vi "Main.vi"(11 "Module Admin":refnum<class "Delacor_lib_QMH_Cloneable Module Admin.lvclass">) -> ()   [LabVIEW 2020, in "NI DAQ.lvlib"]
doc: "This template is based off of the Queued Message Handler design pattern and the Queued Message Handler project template that ships with LabVIEW.\n\nThe main difference is that the queue is private to this module and communication between modules is performed via Broadcast and Request events.\n\nRequest events are wrapped in public API methods and are handled in the Event Handling Loop (EHL) of this VI. Any module can register for Broadcast events sent by this module. The EHL generates messages based on user interface actions.\n\nThe Message Handling Loop (MHL) processes messages generated by the EHL, or by other messages. The messages are string values, so new messages can be added easily to the Message Cases case structure in the MHL. Each message cluster can also provide an optional value for Message Data, which is a variant that can be converted to whatever message-specific data is required.\n_____\nBased on DQMH Project Template 6.1.0.94."
uses:
  NI DAQ.lvlib
  <vilib>/Delacor/Delacor QMH/Libraries/Cloneable Module Admin_class/Delacor_lib_QMH_Cloneable Module Admin.lvclass
  <vilib>/ErrorRing/Error Ring.xnode
  <vilib>/Delacor/Delacor QMH/Libraries/Message Queue_class/Delacor_lib_QMH_Message Queue.lvclass
  Module Data--cluster.ctl
  <vilib>/Utility/miscctls.llb/LVPointTypeDef.ctl
  <vilib>/Utility/error.llb/Error Cluster From Error Code.vi
  <vilib>/Delacor/Delacor QMH/Libraries/Message Queue_class/Delacor_lib_QMH_Enqueue Message (Single).vi
  Stop Argument--cluster.ctl
  Set device ID Argument--cluster.ctl
  Get channel list (Reply Payload)--cluster.ctl
  Get channel list Argument--cluster.ctl
  Start task Argument--cluster.ctl
  Stop task Argument--cluster.ctl
  Write DO Argument--cluster.ctl
  Create DI channel Argument--cluster.ctl
  Read DI (Reply Payload)--cluster.ctl
  Read DI Argument--cluster.ctl
  Support/Task list.ctl
  Get task ref (Reply Payload)--cluster.ctl
  Get task ref Argument--cluster.ctl
  <vilib>/DAQmx/write.llb/DAQmx Write (Digital 1D Bool 1Chan 1Samp).vi
  Create AI channel Argument--cluster.ctl
  Read AI (Reply Payload)--cluster.ctl
  Read AI Argument--cluster.ctl
  Create AO channel Argument--cluster.ctl
  AI config parameters--cluster.ctl
  Write AO Argument--cluster.ctl
  Validate connection Argument--cluster.ctl
  <resource>/objmgr/daqmx.rc
  Validate connection (Reply Payload)--cluster.ctl
  <vilib>/DAQmx/write.llb/DAQmx Write (Digital Bool 1Line 1Point).vi
  <vilib>/DAQmx/write.llb/DAQmx Write (Analog DBL 1Chan 1Samp).vi
  <vilib>/DAQmx/read.llb/DAQmx Read (Analog 1D DBL NChan 1Samp).vi
  <vilib>/DAQmx/read.llb/DAQmx Read (Analog DBL 1Chan 1Samp).vi
  <vilib>/DAQmx/create/channels.llb/DAQmx Create Channel (DO-Digital Output).vi
  <vilib>/DAQmx/create/channels.llb/DAQmx Create Channel (AI-Voltage-Basic).vi
  <vilib>/DAQmx/create/channels.llb/DAQmx Create Channel (DI-Digital Input).vi
  <vilib>/DAQmx/write.llb/DAQmx Write (Analog 1D DBL NChan 1Samp).vi
  Support/Continuous aquisition params.ctl
  Start continous acquisition Argument--cluster.ctl
  Stop continuous acquisition Argument--cluster.ctl
  <vilib>/DAQmx/write.llb/DAQmx Write (Digital 1D Bool NChan 1Samp 1Line).vi
  <vilib>/DAQmx/read.llb/DAQmx Read (Digital 1D Bool 1Chan 1Samp).vi
  <vilib>/DAQmx/read.llb/DAQmx Read (Digital 1D Bool NChan 1Samp 1Line).vi
  Create DO channel Argument--cluster.ctl
  Create CI channel Argument--cluster.ctl
  <vilib>/DAQmx/create/channels.llb/DAQmx Create Channel (CI-Count Edges).vi
  <vilib>/DAQmx/create/channels.llb/DAQmx Create Channel (AO-Voltage-Basic).vi
  Read CI (Reply Payload)--cluster.ctl
  Read CI Argument--cluster.ctl
  <vilib>/DAQmx/read.llb/DAQmx Read (Counter DBL 1Chan 1Samp).vi
  <vilib>/DAQmx/read.llb/DAQmx Read (Counter 1D DBL NChan 1Samp).vi
  <vilib>/DAQmx/read.llb/DAQmx Read (Digital Bool 1Line 1Point).vi
  <vilib>/DAQmx/read.llb/DAQmx Read (Digital 1D U8 1Chan NSamp).vi
panel:
  out "error out":errorcluster
  out "Status":string
  in  "Simulate EHL Error":bool
  in  "Simulate MHL Error":bool
  # "Other QMH Modules communicate with this Module via its Public API (wrappers for its Request Events).\n\nThis Module communicates with other Modules via its Broadcast Events.\nAny module that wants to get these messages, just registers for this module's Broadcast events."
  # "This template is for the Delacor Modified Queued Message Handler design pattern.\n\nSee the block diagram for more information on how to use this template."
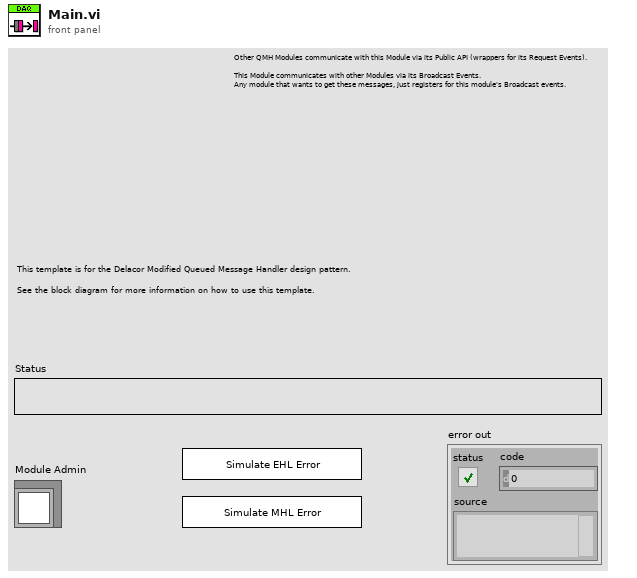
[diagram p1: front panel]
types:
  T1 = typedef "NI DAQ.lvlib/Request Events--cluster.ctl" = cluster{"Stop Module":refnum<user-event>, "Show Panel":refnum<user-event>, "Hide Panel":refnum<user-event>, "Show Diagram":refnum<user-event>, "Get Module Execution Status":refnum<user-event>, "Set device ID":refnum<user-event>, "Get channel list":refnum<user-event>, "Start task":refnum<user-event>, "Stop task":refnum<user-event>, "Write DO":refnum<user-event>, "Create DI channel":refnum<user-event>, "Read DI":refnum<user-event>, "Get task ref":refnum<user-event>, "Wake up HL":refnum<user-event>, "Sleep HL":refnum<user-event>, "Create AI channel":refnum<user-event>, "Read AI":refnum<user-event>, "Create AO channel":refnum<user-event>, "Write AO":refnum<user-event>, "Validate connection":refnum<user-event>, "Start continous acquisition":refnum<user-event>, "Stop continuous acquisition":refnum<user-event>, "Create DO channel":refnum<user-event>, "Create CI channel":refnum<user-event>, "Read CI":refnum<user-event>}
  T2 = cluster{"Wake HL":refnum<user-event>, "Sleep HL":refnum<user-event>}
  T3 = typedef "NI DAQ.lvlib/Continuous aquisition params.ctl" = cluster{"Module ID":i32, "Task list":T4, "Timeout":i32, "Acq type":enum16{"Single", "Multiple"}, "Data in":variant, "DAQmx Task":refnum<k21>, "N samples":i32}
  T4 = typedef "NI DAQ.lvlib/Task list.ctl" = enum16{"All", "DO task", "DI task", "AO task", "AI task", "CI task", "CO task"}
  T5 = typedef "NI DAQ.lvlib/Module Data--cluster.ctl" = cluster{"Status":string, "DO task":refnum<k21>, "DI task":refnum<k21>, "AO task":refnum<k21>, "AI task":refnum<k21>, "Device name":tag, "CI task":refnum<k21>, "CO task":refnum<k21>}
  T6 = enum32{"invalid lock state", "Not Locked", "Locked (No Password)", "Password-protected"}
  T7 = typedef "NI DAQ.lvlib/Stop Argument--cluster.ctl" = cluster{"Module ID":i32, "Origin":string, "Exit via Stop Module Req?":bool, "Wait for Module to stop?":bool}
  T8 = typedef "NI DAQ.lvlib/Set device ID Argument--cluster.ctl" = cluster{"Module ID":i32, "Device ID":tag}
  T9 = typedef "NI DAQ.lvlib/Get channel list Argument--cluster.ctl" = cluster{"Module ID":i32, "Wait Notifier":refnum<notifier>, "wait for reply":bool}
  T10 = typedef "NI DAQ.lvlib/Start task Argument--cluster.ctl" = cluster{"Module ID":i32, "Task list":T4}
  T11 = typedef "NI DAQ.lvlib/Stop task Argument--cluster.ctl" = cluster{"Module ID":i32, "Task list":T4}
  T12 = typedef "NI DAQ.lvlib/Write DO Argument--cluster.ctl" = cluster{"Module ID":i32, "Samples":enum16{"Single", "Multiple"}, "Data":bool[]}
  T13 = typedef "NI DAQ.lvlib/Create DI channel Argument--cluster.ctl" = cluster{"Module ID":i32, "Physical channel":string, "Channel name":string}
  T14 = typedef "NI DAQ.lvlib/Read DI Argument--cluster.ctl" = cluster{"Module ID":i32, "Samples":enum16{"Single", "Multiple"}, "Wait Notifier":refnum<notifier>, "wait for reply":bool}
  T15 = typedef "NI DAQ.lvlib/Get task ref Argument--cluster.ctl" = cluster{"Module ID":i32, "Task list":T4, "Wait Notifier":refnum<notifier>, "wait for reply":bool}
  T16 = typedef "NI DAQ.lvlib/Create AI channel Argument--cluster.ctl" = cluster{"Module ID":i32, "Physical channel":string, "Channel name":string, "Config params":cluster{"input terminal configuration":i32, "minimum value":dbl, "maximum value":dbl}}
  T17 = typedef "NI DAQ.lvlib/Read AI Argument--cluster.ctl" = cluster{"Module ID":i32, "Samples":enum16{"Single", "Multiple"}, "Wait Notifier":refnum<notifier>, "wait for reply":bool}
  T18 = typedef "NI DAQ.lvlib/Create AO channel Argument--cluster.ctl" = cluster{"Module ID":i32, "Physical channel":string, "Channel name":string, "Config params":T19}
  T19 = typedef "NI DAQ.lvlib/AI config parameters--cluster.ctl" = cluster{"Terminal configuration":i32, "min value":dbl, "max value":dbl}
  T20 = typedef "NI DAQ.lvlib/Write AO Argument--cluster.ctl" = cluster{"Module ID":i32, "Value(s)":dbl[], "Samples":enum16{"Single", "Multiple"}}
  T21 = typedef "NI DAQ.lvlib/Validate connection Argument--cluster.ctl" = cluster{"Module ID":i32, "Wait Notifier":refnum<notifier>, "wait for reply":bool}
  T22 = typedef "NI DAQ.lvlib/Start continous acquisition Argument--cluster.ctl" = cluster{"Module ID":i32, "Task list":T4, "Timeout":i32, "Acq type":enum16{"Single", "Multiple"}, "N samples":i32, "Data in":variant}
  T23 = typedef "NI DAQ.lvlib/Stop continuous acquisition Argument--cluster.ctl" = cluster{"Module ID":i32, "Boolean":bool}
  T24 = typedef "NI DAQ.lvlib/Create DO channel Argument--cluster.ctl" = cluster{"Module ID":i32, "lines":tag, "Channel name":string}
  T25 = typedef "NI DAQ.lvlib/Create CI channel Argument--cluster.ctl" = cluster{"Module ID":i32, "Physical channel":string, "Channel name":string, "Channel config":cluster{"Initial count":u32, "Count direction":i32, "Edge":i32}}
  T26 = typedef "NI DAQ.lvlib/Read CI Argument--cluster.ctl" = cluster{"Module ID":i32, "Samples":enum16{"Single", "Multiple"}, "Wait Notifier":refnum<notifier>, "wait for reply":bool}
  T27 = typedef "LVPointTypeDef.ctl" = cluster{"Horizontal":i16, "Vertical":i16}
  T28 = enum32{"Invalid", "Standard", "Closed", "Hidden", "Minimized", "Maximized"}
  T29 = typedef "NI DAQ.lvlib/Get channel list (Reply Payload)--cluster.ctl" = cluster{"Available channels":i32, "error":errorcluster, "Available channels 2":string[][]}
  T30 = typedef "NI DAQ.lvlib/Read DI (Reply Payload)--cluster.ctl" = cluster{"Data":bool[], "error":errorcluster}
  T31 = typedef "NI DAQ.lvlib/Read AI (Reply Payload)--cluster.ctl" = cluster{"Data":dbl[], "error":errorcluster}
  T32 = typedef "NI DAQ.lvlib/Get task ref (Reply Payload)--cluster.ctl" = cluster{"DAQmx Task":refnum<k21>, "error":errorcluster}
  T33 = typedef "NI DAQ.lvlib/Validate connection (Reply Payload)--cluster.ctl" = cluster{"DevSerialNum":u32, "error":errorcluster}
  T34 = typedef "NI DAQ.lvlib/Read CI (Reply Payload)--cluster.ctl" = cluster{"Module ID":i32, "data":dbl[], "error":errorcluster}
  T35 = cluster{"input terminal configuration":i32, "minimum value":dbl, "maximum value":dbl}
  T36 = cluster{"Initial count":u32, "Count direction":i32, "Edge":i32}
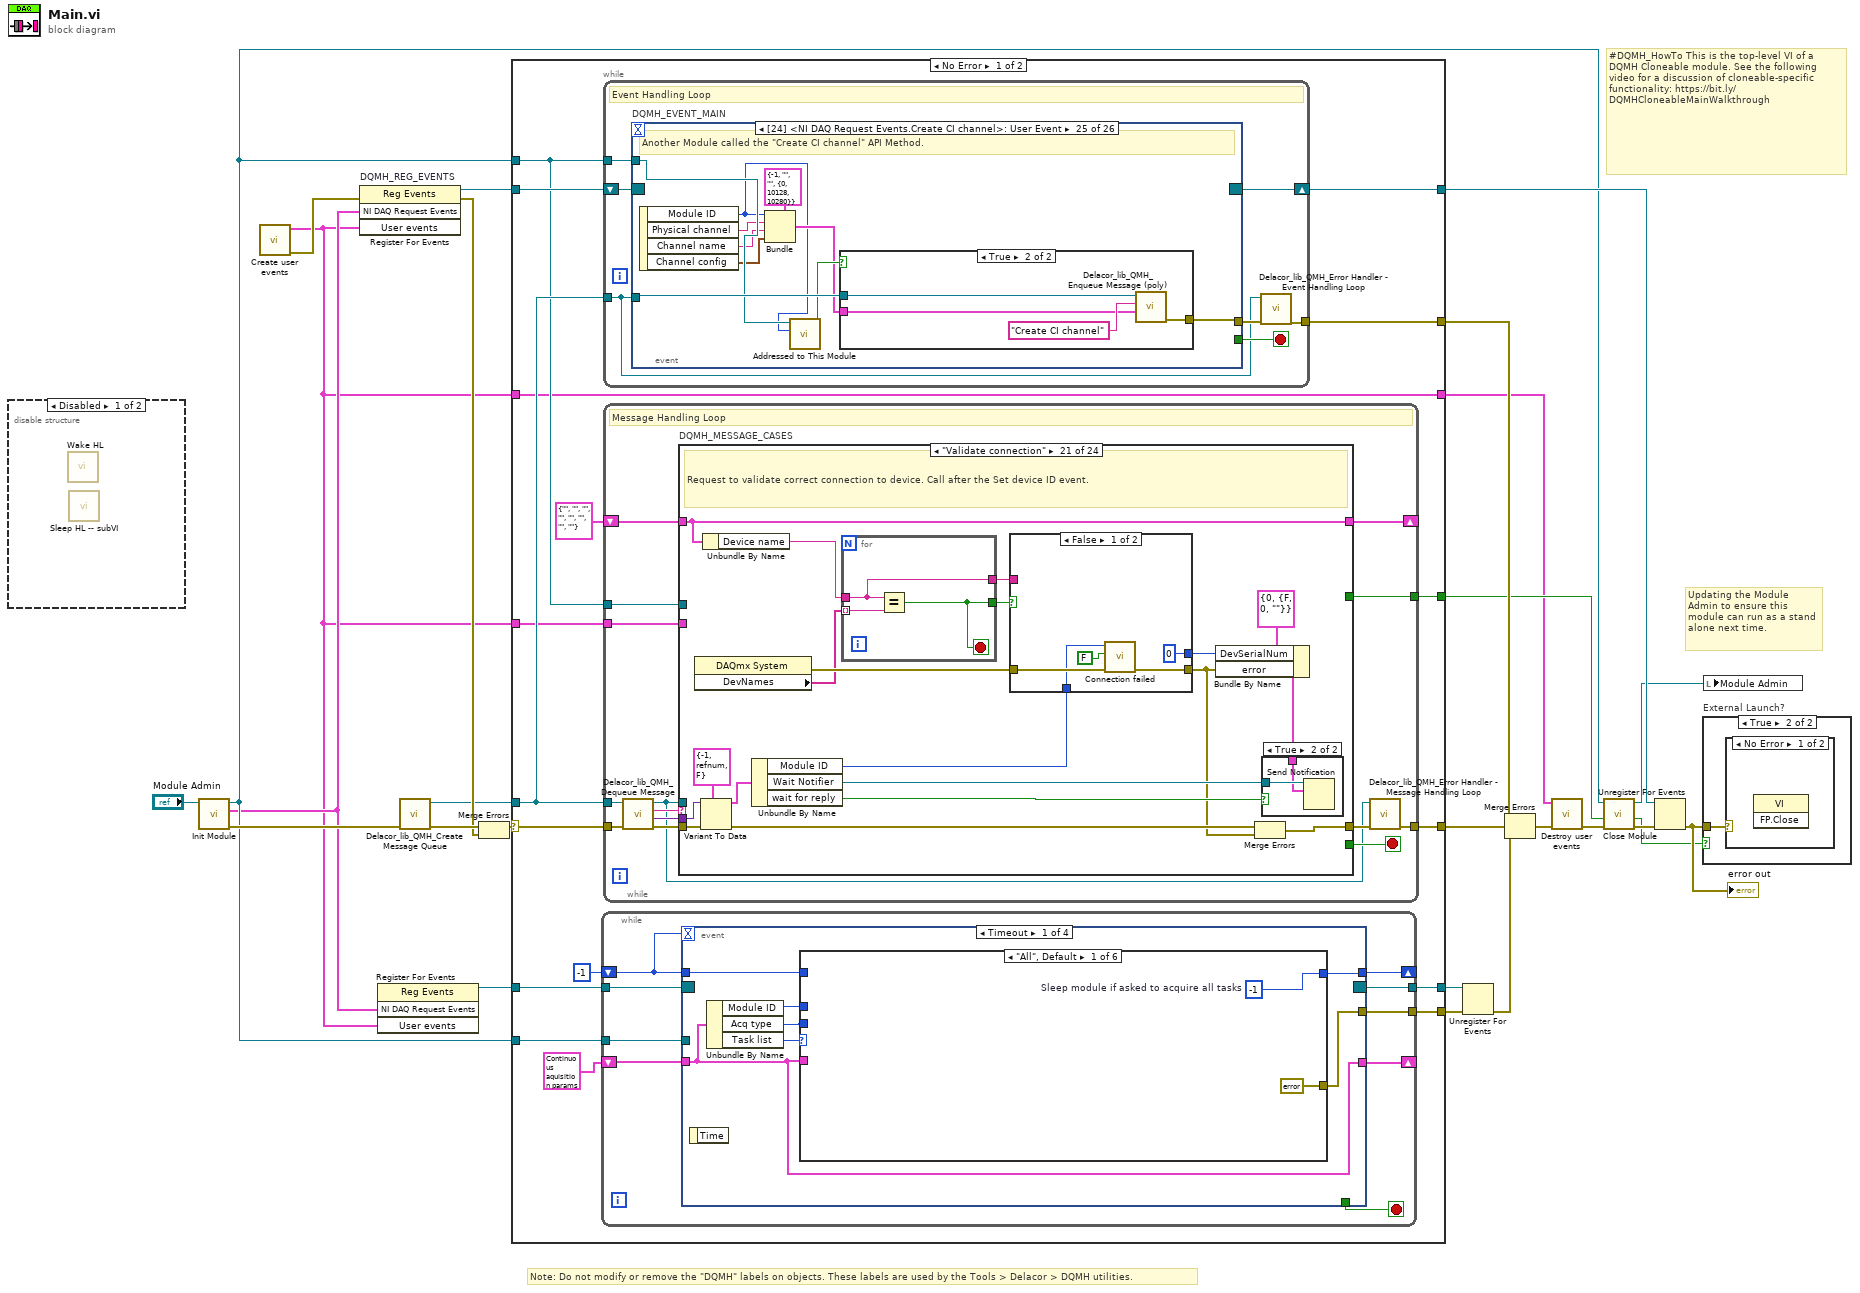
[diagram p0: block diagram]
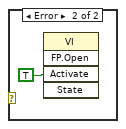
[diagram p4: hidden frame]
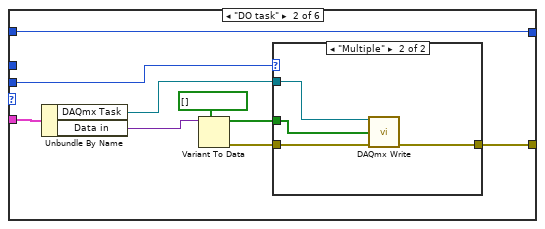
[diagram p5: hidden frame]
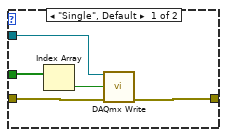
[diagram p6: hidden frame]
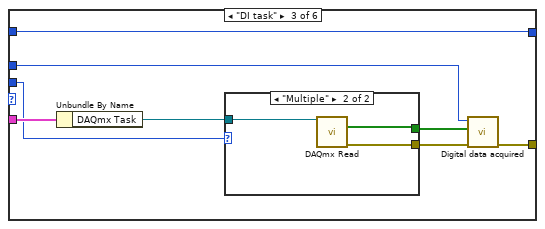
[diagram p7: hidden frame]
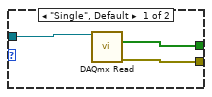
[diagram p8: hidden frame]
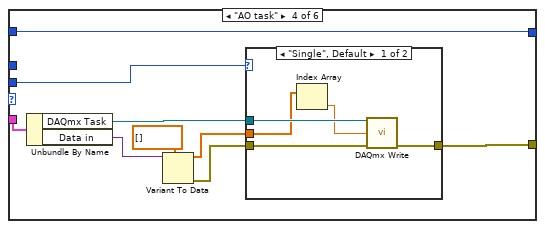
[diagram p9: hidden frame]
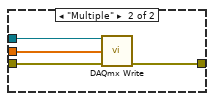
[diagram p10: hidden frame]
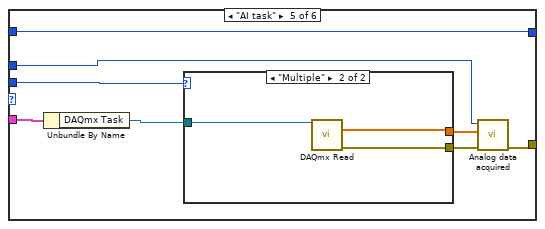
[diagram p11: hidden frame]
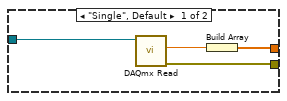
[diagram p12: hidden frame]
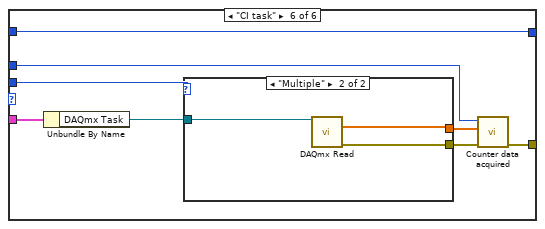
[diagram p13: hidden frame]
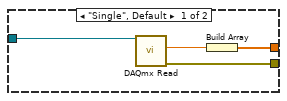
[diagram p14: hidden frame]
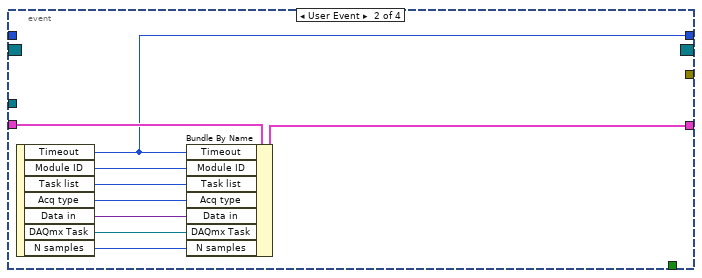
[diagram p15: hidden frame]
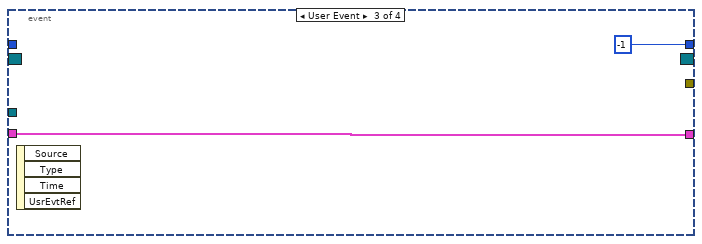
[diagram p16: hidden frame]
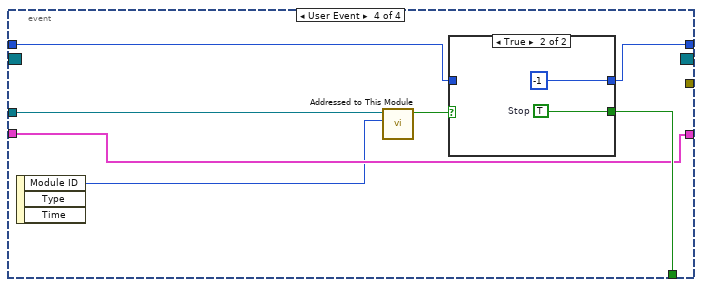
[diagram p17: hidden frame]
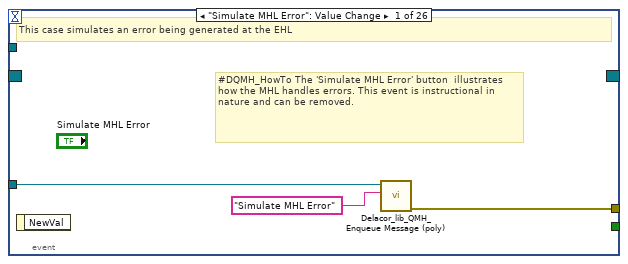
[diagram p19: hidden frame]
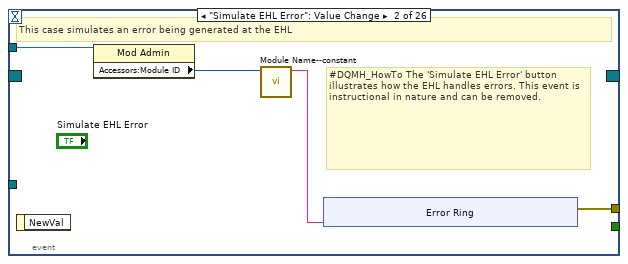
[diagram p20: hidden frame]
diagram:
  # "#DQMH_HowTo This is the top-level VI of a DQMH Cloneable module. See the following video for a discussion of cloneable-specific functionality: https://bit.ly/DQMHCloneableMainWalkthrough"
  # "Note: Do not modify or remove the \"DQMH\" labels on objects. These labels are used by the Tools > Delacor > DQMH utilities."
  # "Updating the Module Admin to ensure this module can run as a stand alone next time."
  n1 = disable-structure shown="Disabled" {
    frame Disabled {
      n2 = call "Wake HL.vi"() -> ()  [unwired: 11 in, 1 out]
      n3 = call "Sleep HL -- subVI.vi"() -> ()  [unwired: 11 in, 1 out]
    }
    frame Enabled {
    }
  }
  n4 = call "Init Module.vi"("Cloneable Module Admin in"="Module Admin") -> ("error out"=w24:errorcluster, "NI DAQ Request Events"=w8:T1, "Cloneable Module Admin out"=w10:refnum<class "Delacor_lib_QMH_Cloneable Module Admin.lvclass">)  [unwired: 8 in]
  n5 = call "Create user events.vi"() -> ("error out"=w9:errorcluster, "User events"=w2:T2)  [unwired: 10 in]
  n6 = register-events "DQMH_REG_EVENTS"(error in=w9, w8, w2) -> (reference out=w17:refnum<event-registration>, error out=w19:errorcluster)  [unwired: 1 in]
  n7 = register-events(w8, w2) -> (reference out=w11:refnum<event-registration>)  [unwired: 2 in, 1 out]
  n8 = call <vilib>:"Delacor_lib_QMH_Create Message Queue.vi"("error in"=w24) -> ("error out"=w21:errorcluster, "Message Queue"=w16:refnum<class "Delacor_lib_QMH_Message Queue.lvclass">)  [unwired: 9 in]
  n9 = Merge Errors(w21, w19) -> (w20:errorcluster)
  n10 = case shown="No Error" w20 {
    selector: w20 -> [w41 w1230]
    tunnel: [w43 w1229] -> w25
    tunnel: [w40 w1237] -> w18
    tunnel: w17 -> [w38 w1237]
    tunnel: w16 -> [w37 w1228]
    tunnel: [w42 _] -> w26
    tunnel: w10 -> [w36 w1233]
    tunnel: [w35 _] -> w13
    tunnel: w11 -> [w34 w1227]
    tunnel: w10 -> [w32 _]
    tunnel: w2 -> [w31 w1226]
    tunnel: [w31 w1226] -> w7
    tunnel: [w30 w1227] -> w4
    tunnel: w2 -> [w28 _]
    tunnel: [w27 _] -> w1
    frame No Error {
      n11 = while {
        tunnel: w34 -> [w52]
        shift-right: [w50] -> _
        shift-left: -1 -> [w46]
        shift-right: [w49] -> _
        shift-left: T3 {"Module ID"=0, "Task list"=enum."All", "Timeout"=0, "Acq type"=enum."Single", "Data in"=variant, "DAQmx Task"="", "N samples"=0} ("event data") -> [w48]
        tunnel: w32 -> [w47]
        tunnel: [w45] -> w30
        tunnel: [w44] -> w27
        stop <- w51 stop-if-true
        n12 = event shown="[0] Timeout" {
          selector: w52 -> [_ _ _ _]
          dyn-events: [_ _ _ _] -> w45
          timeout: w46 -> [_ _ _ _]
          tunnel: [_ _ _ w157] -> w51
          tunnel: [w59 w142 -1 ("Timeout") w158] -> w50
          tunnel: [w56 w143 w152 w154] -> w49
          tunnel: w48 -> [w56 w150 w152 w154]
          tunnel: w47 -> [_ _ _ w159]
          tunnel: w46 -> [w58 _ _ w156]
          tunnel: [w54 _ _ _] -> w44
          event Timeout {
            n13 = event-data() -> ()  [unwired: 1 in, 1 out]
            n14 = Unbundle By Name(w56) -> ("Module ID"=w55:i32, "Acq type"=w53:enum16{"Single", "Multiple"}, "Task list"=w57:T4)
            n15 = case shown="\"All\", Default" w57 {
              tunnel: [w61 w70 w87 w102 w119 w134] -> w59
              tunnel: w58 -> [_ w70 w87 w102 w119 w134]
              tunnel: w56 -> [_ w69 w86 w101 w117 w133]
              tunnel: w55 -> [_ _ w82 _ w112 w128]
              tunnel: [errorcluster {"status"=FALSE, "code"=0, "source"=""} ("error out") w63 w81 w94 w118 w131] -> w54
              tunnel: w53 -> [_ w62 w80 w100 w116 w127]
              frame "All", Default {
                w61 = -1  # Sleep module if asked to acquire all tasks
              }
              frame "DO task" {
                n16 = Unbundle By Name(w69) -> ("DAQmx Task"=w68:refnum<k21>, "Data in"=w66:variant)
                n17 = Variant To Data(type=bool[] [], Variant=w66) -> (data=w64:bool[], error out=w67:errorcluster)  [unwired: 1 in]
                n18 = case shown="\"Multiple\"" w62 {
                  tunnel: w68 -> [w75 w76]
                  tunnel: w67 -> [w74 w79]
                  tunnel: w64 -> [w72 w77]
                  tunnel: [w73 w78] -> w63
                  frame "Single", Default {
                    n19 = Index Array(array=w72) -> (element=w71:bool)  [unwired: 1 in]
                    n20 = call-poly <vilib>:"DAQmx Write.vi"("task/channels in"=w75, "data"=w71, "error in"=w74) -> ("error out"=w73:errorcluster)  [unwired: 10 in, 2 out]
                  }
                  frame "Multiple" {
                    n21 = call-poly <vilib>:"DAQmx Write.vi"("task/channels in"=w76, "data"=w77, "error in"=w79) -> ("error out"=w78:errorcluster)  [unwired: 10 in, 2 out]
                  }
                }
              }
              frame "DI task" {
                n22 = Unbundle By Name(w86) -> ("DAQmx Task"=w85:refnum<k21>)
                n23 = case shown="\"Multiple\"" w80 {
                  tunnel: w85 -> [w90 w91]
                  tunnel: [w89 w92] -> w84
                  tunnel: [w88 w93] -> w83
                  frame "Single", Default {
                    n24 = call-poly <vilib>:"DAQmx Read.vi"("task/channels in"=w90) -> ("data"=w89:bool[], "error out"=w88:errorcluster)  [unwired: 12 in, 1 out]
                  }
                  frame "Multiple" {
                    n25 = call-poly <vilib>:"DAQmx Read.vi"("task/channels in"=w91) -> ("data"=w92:bool[], "error out"=w93:errorcluster)  [unwired: 12 in, 1 out]
                  }
                }
                n26 = call "Digital data acquired.vi"("error in"=w83, "Data"=w84, "Module ID"=w82) -> ("error out"=w81:errorcluster)  [unwired: 8 in]
              }
              frame "AO task" {
                n27 = Unbundle By Name(w101) -> ("DAQmx Task"=w99:refnum<k21>, "Data in"=w98:variant)
                n28 = Variant To Data(type=dbl[] [], Variant=w98) -> (data=w95:dbl[], error out=w97:errorcluster)  [unwired: 1 in]
                n29 = case shown="\"Single\", Default" w100 {
                  tunnel: w99 -> [w107 w109]
                  tunnel: [w106 w111] -> w94
                  tunnel: w97 -> [w105 w110]
                  tunnel: w95 -> [w104 w108]
                  frame "Single", Default {
                    n30 = Index Array(array=w104) -> (element=w103:dbl)  [unwired: 1 in]
                    n31 = call-poly <vilib>:"DAQmx Write.vi"("task/channels in"=w107, "data"=w103, "error in"=w105) -> ("error out"=w106:errorcluster)  [unwired: 10 in, 2 out]
                  }
                  frame "Multiple" {
                    n32 = call-poly <vilib>:"DAQmx Write.vi"("task/channels in"=w109, "data"=w108, "error in"=w110) -> ("error out"=w111:errorcluster)  [unwired: 10 in, 2 out]
                  }
                }
              }
              frame "AI task" {
                n33 = Unbundle By Name(w117) -> ("DAQmx Task"=w115:refnum<k21>)
                n34 = case shown="\"Multiple\"" w116 {
                  tunnel: w115 -> [w123 w126]
                  tunnel: [w120 w125] -> w114
                  tunnel: [w122 w124] -> w113
                  frame "Single", Default {
                    n35 = call-poly <vilib>:"DAQmx Read.vi"("task/channels in"=w123) -> ("data"=w121:dbl, "error out"=w122:errorcluster)  [unwired: 12 in, 1 out]
                    n36 = Build Array(w121) -> (w120:dbl[])
                  }
                  frame "Multiple" {
                    n37 = call-poly <vilib>:"DAQmx Read.vi"("task/channels in"=w126) -> ("data"=w125:dbl[], "error out"=w124:errorcluster)  [unwired: 12 in, 1 out]
                  }
                }
                n38 = call "Analog data acquired.vi"("error in"=w113, "Data"=w114, "Module ID"=w112) -> ("error out"=w118:errorcluster)  [unwired: 8 in]
              }
              frame "CI task" {
                n39 = Unbundle By Name(w133) -> ("DAQmx Task"=w132:refnum<k21>)
                n40 = case shown="\"Multiple\"" w127 {
                  tunnel: w132 -> [w138 w141]
                  tunnel: [w135 w140] -> w129
                  tunnel: [w137 w139] -> w130
                  frame "Single", Default {
                    n41 = call-poly <vilib>:"DAQmx Read.vi"("task/channels in"=w138) -> ("data"=w136:dbl, "error out"=w137:errorcluster)  [unwired: 12 in, 1 out]
                    n42 = Build Array(w136) -> (w135:dbl[])
                  }
                  frame "Multiple" {
                    n43 = call-poly <vilib>:"DAQmx Read.vi"("task/channels in"=w141) -> ("data"=w140:dbl[], "error out"=w139:errorcluster)  [unwired: 12 in, 1 out]
                  }
                }
                n44 = call "Counter data acquired.vi"("error in"=w130, "Data"=w129, "Module ID"=w128) -> ("error out"=w131:errorcluster)  [unwired: 8 in]
              }
            }
          }
          event User Event {
            n45 = event-data() -> ("Timeout"=w142:i32, "Module ID"=w144:i32, "Task list"=w145:T4, "Acq type"=w146:enum16{"Single", "Multiple"}, "Data in"=w147:variant, "DAQmx Task"=w148:refnum<k21>, "N samples"=w149:i32)  [unwired: 1 in]
            n46 = Bundle By Name(cluster=w150, "Timeout"=w142, "Module ID"=w144, "Task list"=w145, "Acq type"=w146, "Data in"=w147, "DAQmx Task"=w148, "N samples"=w149) -> (w143:T3)
          }
          event User Event {
            n47 = event-data() -> ()  [unwired: 1 in, 4 out]
          }
          event User Event {
            n48 = event-data() -> ("Module ID"=w153:i32)  [unwired: 1 in, 2 out]
            n49 = call "Addressed to This Module.vi"("Module ID from Argument"=w153, "Module Admin"=w159) -> ("Addressed to this instance?"=w155:bool)  [unwired: 8 in, 1 out]
            n50 = case shown="True" w155 {
              tunnel: [w160 -1] -> w158
              tunnel: [_ w161] -> w157
              tunnel: w156 -> [w160 _]
              frame False {
              }
              frame True {
                w161 = TRUE  # Stop
              }
            }
          }
        }
      }
      n51 = while {
        tunnel: w37 -> [w163]
        shift-right: [w166] -> w40
        shift-left: w38 -> [w167]
        tunnel: [w168] -> w42
        tunnel: w36 -> [w164]
        stop <- w165 stop-if-true
        # "Event Handling Loop"
        n52 = event "DQMH_EVENT_MAIN" shown="[24] <NI DAQ Request Events.Create CI channel>: User Event" {
          selector: w167 -> [_ _ _ _ _ _ _ _ _ _ _ _ _ _ _ _ _ _ _ _ _ _ _ _ _ _]
          dyn-events: [_ _ _ _ _ _ _ _ _ _ _ _ _ _ _ _ _ _ _ _ _ _ _ _ _ _] -> w166
          timeout: _ -> [_ _ _ _ _ _ _ _ _ _ _ _ _ _ _ _ _ _ _ _ _ _ _ _ _ _]
          tunnel: [_ _ _ _ _ _ w224 _ _ _ _ _ _ _ _ _ _ _ _ _ _ _ _ _ _ _] -> w165
          tunnel: w163 -> [w171 _ _ _ _ _ w227 w243 w259 w272 w284 w296 w309 w322 w336 w350 w364 w378 w392 w405 w418 w433 w445 w458 w472 w486]
          tunnel: [w172 w176 _ _ w201 _ w228 w246 w252 w266 w277 w290 w302 w314 w327 w341 w357 w369 w384 w398 w412 w423 w438 w450 w463 w477] -> w169
          tunnel: w164 -> [_ w175 w184 w191 w199 w205 w226 w244 w257 w270 w282 w294 w307 w320 w334 w348 w362 w376 w390 w403 w416 w431 w443 w456 w470 w484]
          event "Simulate MHL Error": Value Change {
            # "#DQMH_HowTo The 'Simulate MHL Error' button  illustrates how the MHL handles errors. This event is instructional in nature and can be removed."
            # "This case simulates an error being generated at the EHL"
            n53 = event-data() -> ()  [unwired: 1 in, 1 out]
            n54 = call-poly <vilib>:"Delacor_lib_QMH_Enqueue Message (poly).vi"("Message"="Simulate MHL Error", "Message Queue in"=w171) -> ("error out"=w172:errorcluster)  [unwired: 8 in, 1 out]
          }
          event "Simulate EHL Error": Value Change {
            # "#DQMH_HowTo The 'Simulate EHL Error' button  illustrates how the EHL handles errors. This event is instructional in nature and can be removed."
            # "This case simulates an error being generated at the EHL"
            n55 = event-data() -> ()  [unwired: 1 in, 1 out]
            n56 = property class="Mod Admin"(reference=w175) -> ("Accessors:Module ID"=w174:i32)  [unwired: 1 in, 2 out]
            n57 = call "Module Name--constant.vi"("Module ID"=w174) -> ("Module Name"=w173:string)  [unwired: 10 in]
            n58 = xnode "Error Ring"("parameter 0"=w173) -> ("error out"=w176:errorcluster)
          }
          event User Event {
            # "Another Module called the \"Show Panel\" API Method."
            n59 = event-data() -> ("Module ID"=w185:i32)  [unwired: 1 in]
            n60 = call "Addressed to This Module.vi"("Module ID from Argument"=w185, "Module Admin"=w184) -> ("Addressed to this instance?"=w186:bool)  [unwired: 8 in, 1 out]
            n61 = case shown="True" w186 {
              tunnel: w184 -> [_ w188]
              frame False {
              }
              frame True {
                # "Show the panel of this VI, and send a status updated message to let listeners know."
                n62 = property class="Mod Admin"(reference=w188) -> ("Accessors:Module ID"=w187:i32)  [unwired: 1 in, 2 out]
                n63 = control-ref of="This VI"() -> (w190:refnum<vi>)
                n64 = call "Open VI Panel.vi"("VI"=w190) -> ()  [unwired: 10 in, 1 out]
                n65 = call "Status Updated.vi"("Status"="Panel shown." ("format string"), "Module ID"=w187) -> ()  [unwired: 9 in, 1 out]
              }
            }
          }
          event User Event {
            # "Another Module called the \"Hide Panel\" API Method."
            n66 = event-data() -> ("Module ID"=w192:i32)  [unwired: 1 in]
            n67 = call "Addressed to This Module.vi"("Module ID from Argument"=w192, "Module Admin"=w191) -> ("Addressed to this instance?"=w193:bool)  [unwired: 8 in, 1 out]
            n68 = case shown="True" w193 {
              tunnel: w191 -> [_ w195]
              frame False {
              }
              frame True {
                # "Hide the panel of this VI, and send a status updated message to let listeners know."
                n69 = property class="Mod Admin"(reference=w195) -> ("Accessors:Module ID"=w194:i32)  [unwired: 1 in, 2 out]
                n70 = control-ref of="This VI"() -> (w197:refnum<vi>)
                n71 = call "Hide VI Panel.vi"("VI"=w197) -> ()  [unwired: 10 in, 1 out]
                n72 = call "Status Updated.vi"("Status"="Panel hidden." ("format string"), "Module ID"=w194) -> ()  [unwired: 9 in, 1 out]
              }
            }
          }
          event User Event {
            # "For cloneable running as singleton, broadcast that the module is running."
            n73 = event-data() -> ("Module ID"=w198:i32)  [unwired: 1 in]
            n74 = call "Addressed to This Module.vi"("Module ID from Argument"=w198, "Module Admin"=w199) -> ("Addressed to this instance?"=w200:bool)  [unwired: 8 in, 1 out]
            n75 = case shown="True" w200 {
              tunnel: [_ w204] -> w201
              tunnel: w198 -> [_ w203]
              frame False {
              }
              frame True {
                n76 = call "Update Module Execution Status.vi"("Running?"=TRUE, "Module ID"=w203) -> ("error out"=w204:errorcluster)  [unwired: 9 in]
              }
            }
          }
          event User Event {
            # "Another Module called the \"Show Diagram\" API Method. This event is used for debugging."
            n77 = event-data() -> ("Module ID"=w206:i32)  [unwired: 1 in]
            n78 = call "Addressed to This Module.vi"("Module ID from Argument"=w206, "Module Admin"=w205) -> ("Addressed to this instance?"=w207:bool)  [unwired: 8 in, 1 out]
            n79 = case shown="True" w207 {
              tunnel: w205 -> [_ w208]
              frame False {
              }
              frame True {
                n80 = disable-structure shown="RUN_TIME_ENGINE==False" {
                  disable-tunnel: w208 -> [w209 _]
                  frame condition #0 (active) {
                    # "functionality not available in exe"
                    n81 = invoke class="VI" method="Lock State.Get"() -> (error out=w215:errorcluster, "Get Lock State"=w214:T6, "pwd in cache"=w211:bool)  [unwired: 4 in, 1 out]
                    n82 = Equal?(x=T6."Password-protected", y=w214) -> (x = y?=w212:bool)
                    n83 = Compound Arithmetic op=AND(w212, invert w211) -> (w210:bool)
                    n84 = case shown="False" w210 {
                      tunnel: w215 -> [w220 _]
                      tunnel: w209 -> [w217 _]
                      frame False {
                        n85 = property class="Mod Admin"(reference=w217) -> ("Accessors:Module ID"=w216:i32)  [unwired: 1 in, 2 out]
                        n86 = property class="VI"(error in=w220, "BDWin.Open"=TRUE ("Block Diagram Window:Open")) -> ()  [unwired: 1 in, 2 out]
                        n87 = call "Status Updated.vi"("Status"="Block Diagram shown." ("format string"), "Module ID"=w216) -> ()  [unwired: 9 in, 1 out]
                      }
                      frame True {
                        # "Password-protected VI, and the password is not in the cache. Do not show the diagram."
                      }
                    }
                  }
                  frame condition #1 {
                  }
                }
              }
            }
          }
          event User Event {
            # "Another Module called the \"Stop Module\" API Method  or the Message Handling Loop below."
            n88 = event-data() -> ("Module ID"=w222:i32, "Wait for Module to stop?"=w223:bool, "Origin"=w221:string)  [unwired: 1 in]
            n89 = call "Addressed to This Module.vi"("Module ID from Argument"=w222, "Module Admin"=w226) -> ("Addressed to this instance?"=w225:bool)  [unwired: 8 in, 1 out]
            n90 = case shown="True" w225 {
              tunnel: [_ w240] -> w228
              tunnel: w227 -> [_ w236]
              tunnel: [_ TRUE] -> w224
              tunnel: w223 -> [_ w231]
              tunnel: w222 -> [_ w233]
              tunnel: w221 -> [_ w229]
              frame False {
              }
              frame True {
                # "The event can get fired from the Exit message. The queue gets destroyed there. In this case, the Enqueue VI will return error 1. It is safe to ignore, because the module is already exiting."
                n91 = local write "Status"(w229) -> ()
                n92 = Bundle By Name(cluster=T7 {"Module ID"=-1, "Origin"="", "Exit via Stop Module Req?"=FALSE, "Wait for Module to stop?"=FALSE} ("Stop Argument"), "Module ID"=w233, "Exit via Stop Module Req?"=TRUE, "Wait for Module to stop?"=w231) -> (w230:T7)
                n93 = call-poly <vilib>:"Delacor_lib_QMH_Enqueue Message (poly).vi"("Priority Message? (F)"=TRUE, "Message Data"=w230, "Message"="Exit", "Message Queue in"=w236) -> ("error out"=w241:errorcluster)  [unwired: 6 in, 1 out]
                n94 = call <vilib>:"Clear Errors.vi"("error in (no error)"=w241, "specific error code to clear (0: all)"=1) -> ("error out"=w240:errorcluster)  [unwired: 4 in, 1 out]
              }
            }
          }
          event Panel Close? {
            w245 = TRUE  # Discard the event, the MHL is responsible for closing and stopping this VI.
            # "Hide the panel or send the 'Exit' message if the user clicks the 'X' on the module main VI panel."
            n95 = event-data() -> ()  [unwired: 1 in, 1 out]
            n96 = property class="Mod Admin"(reference=w244) -> ("Accessors:External Launch"=w242:bool)  [unwired: 1 in, 2 out]
            n97 = case shown="True" w242 {
              tunnel: w243 -> [_ w250]
              tunnel: [_ w251] -> w246
              frame True {
                # "If externally launched, clicking the 'X' hides the panel, but doesn't close it."
                n98 = control-ref of="This VI"() -> (w247:refnum<vi>)
                n99 = call "Hide VI Panel.vi"("VI"=w247) -> ()  [unwired: 10 in, 1 out]
              }
              frame False {
                # "If run as a stand-alone VI, clicking the panel 'X' stops the VI."
                n100 = call-poly <vilib>:"Delacor_lib_QMH_Enqueue Message (poly).vi"("Priority Message? (F)"=TRUE, "Message"="Exit", "Message Queue in"=w250) -> ("error out"=w251:errorcluster)  [unwired: 7 in, 1 out]
              }
            }
            n101 = event-data("Discard?"=w245) -> ()  [unwired: 1 in, 1 out]
          }
          event User Event {
            # "Another Module called the \"Set device ID\" API Method."
            n102 = event-data() -> ("Module ID"=w254:i32, "Device ID"=w253:tag)  [unwired: 1 in]
            n103 = Bundle(cluster=T8 {"Module ID"=-1, "Device ID"=""} ("Set device ID Argument"), "Module ID"=w254, "Device ID"=w253) -> (w255:T8)
            n104 = call "Addressed to This Module.vi"("Module ID from Argument"=w254, "Module Admin"=w257) -> ("Addressed to this instance?"=w258:bool)  [unwired: 8 in, 1 out]
            n105 = case shown="True" w258 {
              tunnel: w259 -> [_ w263]
              tunnel: w255 -> [_ w261]
              tunnel: [_ w260] -> w252
              frame False {
              }
              frame True {
                n106 = call-poly <vilib>:"Delacor_lib_QMH_Enqueue Message (poly).vi"("Message Data"=w261, "Message"="Set device ID", "Message Queue in"=w263) -> ("error out"=w260:errorcluster)  [unwired: 7 in, 1 out]
              }
            }
          }
          event User Event {
            # "Another Module called the \"Get channel list\" API Method."
            n107 = event-data() -> ("Module ID"=w267:i32, "Wait Notifier"=w265:refnum<notifier>, "wait for reply"=w264:bool)  [unwired: 1 in]
            n108 = Bundle(cluster=T9 {"Module ID"=-1, "Wait Notifier"=refnum, "wait for reply"=FALSE} ("Get channel list Argument"), "Module ID"=w267, "Wait Notifier"=w265, "wait for reply"=w264) -> (w268:T9)
            n109 = call "Addressed to This Module.vi"("Module ID from Argument"=w267, "Module Admin"=w270) -> ("Addressed to this instance?"=w271:bool)  [unwired: 8 in, 1 out]
            n110 = case shown="True" w271 {
              tunnel: w272 -> [_ w276]
              tunnel: w268 -> [_ w274]
              tunnel: [_ w273] -> w266
              frame False {
              }
              frame True {
                n111 = call-poly <vilib>:"Delacor_lib_QMH_Enqueue Message (poly).vi"("Message Data"=w274, "Message"="Get channel list", "Message Queue in"=w276) -> ("error out"=w273:errorcluster)  [unwired: 7 in, 1 out]
              }
            }
          }
          event User Event {
            # "Another Module called the \"Start task\" API Method."
            n112 = event-data() -> ("Module ID"=w279:i32, "Task list"=w278:T4)  [unwired: 1 in]
            n113 = Bundle(cluster=T10 {"Module ID"=-1, "Task list"=enum."All"} ("Start task Argument"), "Module ID"=w279, "Task list"=w278) -> (w280:T10)
            n114 = call "Addressed to This Module.vi"("Module ID from Argument"=w279, "Module Admin"=w282) -> ("Addressed to this instance?"=w283:bool)  [unwired: 8 in, 1 out]
            n115 = case shown="True" w283 {
              tunnel: w284 -> [_ w288]
              tunnel: w280 -> [_ w286]
              tunnel: [_ w285] -> w277
              frame False {
              }
              frame True {
                n116 = call-poly <vilib>:"Delacor_lib_QMH_Enqueue Message (poly).vi"("Message Data"=w286, "Message"="Start task", "Message Queue in"=w288) -> ("error out"=w285:errorcluster)  [unwired: 7 in, 1 out]
              }
            }
          }
          event User Event {
            # "Another Module called the \"Stop task\" API Method."
            n117 = event-data() -> ("Module ID"=w291:i32, "Task list"=w289:T4)  [unwired: 1 in]
            n118 = Bundle(cluster=T11 {"Module ID"=-1, "Task list"=enum."All"} ("Stop task Argument"), "Module ID"=w291, "Task list"=w289) -> (w292:T11)
            n119 = call "Addressed to This Module.vi"("Module ID from Argument"=w291, "Module Admin"=w294) -> ("Addressed to this instance?"=w295:bool)  [unwired: 8 in, 1 out]
            n120 = case shown="True" w295 {
              tunnel: w296 -> [_ w300]
              tunnel: w292 -> [_ w298]
              tunnel: [_ w297] -> w290
              frame False {
              }
              frame True {
                n121 = call-poly <vilib>:"Delacor_lib_QMH_Enqueue Message (poly).vi"("Message Data"=w298, "Message"="Stop task", "Message Queue in"=w300) -> ("error out"=w297:errorcluster)  [unwired: 7 in, 1 out]
              }
            }
          }
          event User Event {
            # "Another Module called the \"Write DO\" API Method."
            n122 = event-data() -> ("Module ID"=w304:i32, "Samples"=w303:enum16{"Single", "Multiple"}, "Data"=w301:bool[])  [unwired: 1 in]
            n123 = Bundle(cluster=T12 {"Module ID"=-1, "Samples"=enum."Single", "Data"=[]} ("Write DO Argument"), "Module ID"=w304, "Samples"=w303, "Data"=w301) -> (w305:T12)
            n124 = call "Addressed to This Module.vi"("Module ID from Argument"=w304, "Module Admin"=w307) -> ("Addressed to this instance?"=w308:bool)  [unwired: 8 in, 1 out]
            n125 = case shown="True" w308 {
              tunnel: w309 -> [_ w313]
              tunnel: w305 -> [_ w311]
              tunnel: [_ w310] -> w302
              frame False {
              }
              frame True {
                n126 = call-poly <vilib>:"Delacor_lib_QMH_Enqueue Message (poly).vi"("Message Data"=w311, "Message"="Write DO", "Message Queue in"=w313) -> ("error out"=w310:errorcluster)  [unwired: 7 in, 1 out]
              }
            }
          }
          event User Event {
            # "Another Module called the \"Create DI channel\" API Method."
            n127 = event-data() -> ("Module ID"=w317:i32, "Physical channel"=w316:string, "Channel name"=w315:string)  [unwired: 1 in]
            n128 = Bundle(cluster=T13 {"Module ID"=-1, "Physical channel"="", "Channel name"=""} ("Create DI channel Argument"), "Module ID"=w317, "Physical channel"=w316, "Channel name"=w315) -> (w318:T13)
            n129 = call "Addressed to This Module.vi"("Module ID from Argument"=w317, "Module Admin"=w320) -> ("Addressed to this instance?"=w321:bool)  [unwired: 8 in, 1 out]
            n130 = case shown="True" w321 {
              tunnel: w322 -> [_ w326]
              tunnel: w318 -> [_ w324]
              tunnel: [_ w323] -> w314
              frame False {
              }
              frame True {
                n131 = call-poly <vilib>:"Delacor_lib_QMH_Enqueue Message (poly).vi"("Message Data"=w324, "Message"="Create DI channel", "Message Queue in"=w326) -> ("error out"=w323:errorcluster)  [unwired: 7 in, 1 out]
              }
            }
          }
          event User Event {
            # "Another Module called the \"Read DI\" API Method."
            n132 = event-data() -> ("Module ID"=w331:i32, "Samples"=w330:enum16{"Single", "Multiple"}, "Wait Notifier"=w329:refnum<notifier>, "wait for reply"=w328:bool)  [unwired: 1 in]
            n133 = Bundle(cluster=T14 {"Module ID"=-1, "Samples"=enum."Single", "Wait Notifier"=refnum, "wait for reply"=FALSE} ("Read DI Argument"), "Module ID"=w331, "Samples"=w330, "Wait Notifier"=w329, "wait for reply"=w328) -> (w332:T14)
            n134 = call "Addressed to This Module.vi"("Module ID from Argument"=w331, "Module Admin"=w334) -> ("Addressed to this instance?"=w335:bool)  [unwired: 8 in, 1 out]
            n135 = case shown="True" w335 {
              tunnel: w336 -> [_ w340]
              tunnel: w332 -> [_ w338]
              tunnel: [_ w337] -> w327
              frame False {
              }
              frame True {
                n136 = call-poly <vilib>:"Delacor_lib_QMH_Enqueue Message (poly).vi"("Message Data"=w338, "Message"="Read DI", "Message Queue in"=w340) -> ("error out"=w337:errorcluster)  [unwired: 7 in, 1 out]
              }
            }
          }
          event User Event {
            # "Another Module called the \"Get task ref\" API Method."
            n137 = event-data() -> ("Module ID"=w345:i32, "Task list"=w344:T4, "Wait Notifier"=w343:refnum<notifier>, "wait for reply"=w342:bool)  [unwired: 1 in]
            n138 = Bundle(cluster=T15 {"Module ID"=-1, "Task list"=enum."All", "Wait Notifier"=refnum, "wait for reply"=FALSE} ("Get task ref Argument"), "Module ID"=w345, "Task list"=w344, "Wait Notifier"=w343, "wait for reply"=w342) -> (w346:T15)
            n139 = call "Addressed to This Module.vi"("Module ID from Argument"=w345, "Module Admin"=w348) -> ("Addressed to this instance?"=w349:bool)  [unwired: 8 in, 1 out]
            n140 = case shown="True" w349 {
              tunnel: w350 -> [_ w354]
              tunnel: w346 -> [_ w352]
              tunnel: [_ w351] -> w341
              frame False {
              }
              frame True {
                n141 = call-poly <vilib>:"Delacor_lib_QMH_Enqueue Message (poly).vi"("Message Data"=w352, "Message"="Get task ref", "Message Queue in"=w354) -> ("error out"=w351:errorcluster)  [unwired: 7 in, 1 out]
              }
            }
          }
          event User Event {
            # "Another Module called the \"Create AI channel\" API Method."
            n142 = event-data() -> ("Module ID"=w359:i32, "Physical channel"=w358:string, "Channel name"=w356:string, "Config params"=w355:T35)  [unwired: 1 in]
            n143 = Bundle(cluster=T16 {"Module ID"=-1, "Physical channel"="", "Channel name"="", "Config params"={"input terminal configuration"=-1, "minimum value"=-5.0, "maximum value"=5.0}} ("Create AI channel Argument"), "Module ID"=w359, "Physical channel"=w358, "Channel name"=w356, "Config params"=w355) -> (w360:T16)
            n144 = call "Addressed to This Module.vi"("Module ID from Argument"=w359, "Module Admin"=w362) -> ("Addressed to this instance?"=w363:bool)  [unwired: 8 in, 1 out]
            n145 = case shown="True" w363 {
              tunnel: w364 -> [_ w368]
              tunnel: w360 -> [_ w366]
              tunnel: [_ w365] -> w357
              frame False {
              }
              frame True {
                n146 = call-poly <vilib>:"Delacor_lib_QMH_Enqueue Message (poly).vi"("Message Data"=w366, "Message"="Create AI channel", "Message Queue in"=w368) -> ("error out"=w365:errorcluster)  [unwired: 7 in, 1 out]
              }
            }
          }
          event User Event {
            # "Another Module called the \"Read AI\" API Method."
            n147 = event-data() -> ("Module ID"=w373:i32, "Samples"=w372:enum16{"Single", "Multiple"}, "Wait Notifier"=w371:refnum<notifier>, "wait for reply"=w370:bool)  [unwired: 1 in]
            n148 = Bundle(cluster=T17 {"Module ID"=-1, "Samples"=enum."Single", "Wait Notifier"=refnum, "wait for reply"=FALSE} ("Read AI Argument"), "Module ID"=w373, "Samples"=w372, "Wait Notifier"=w371, "wait for reply"=w370) -> (w374:T17)
            n149 = call "Addressed to This Module.vi"("Module ID from Argument"=w373, "Module Admin"=w376) -> ("Addressed to this instance?"=w377:bool)  [unwired: 8 in, 1 out]
            n150 = case shown="True" w377 {
              tunnel: w378 -> [_ w382]
              tunnel: w374 -> [_ w380]
              tunnel: [_ w379] -> w369
              frame False {
              }
              frame True {
                n151 = call-poly <vilib>:"Delacor_lib_QMH_Enqueue Message (poly).vi"("Message Data"=w380, "Message"="Read AI", "Message Queue in"=w382) -> ("error out"=w379:errorcluster)  [unwired: 7 in, 1 out]
              }
            }
          }
          event User Event {
            # "Another Module called the \"Create AO channel\" API Method."
            n152 = event-data() -> ("Module ID"=w387:i32, "Physical channel"=w386:string, "Channel name"=w385:string, "Config params"=w383:T19)  [unwired: 1 in]
            n153 = Bundle(cluster=T18 {"Module ID"=-1, "Physical channel"="", "Channel name"="", "Config params"={"Terminal configuration"=-1, "min value"=-5.0, "max value"=5.0}} ("Create AO channel Argument"), "Module ID"=w387, "Physical channel"=w386, "Channel name"=w385, "Config params"=w383) -> (w388:T18)
            n154 = call "Addressed to This Module.vi"("Module ID from Argument"=w387, "Module Admin"=w390) -> ("Addressed to this instance?"=w391:bool)  [unwired: 8 in, 1 out]
            n155 = case shown="True" w391 {
              tunnel: w392 -> [_ w396]
              tunnel: w388 -> [_ w394]
              tunnel: [_ w393] -> w384
              frame False {
              }
              frame True {
                n156 = call-poly <vilib>:"Delacor_lib_QMH_Enqueue Message (poly).vi"("Message Data"=w394, "Message"="Create AO channel", "Message Queue in"=w396) -> ("error out"=w393:errorcluster)  [unwired: 7 in, 1 out]
              }
            }
          }
          event User Event {
            # "Another Module called the \"Write AO\" API Method."
            n157 = event-data() -> ("Module ID"=w400:i32, "Value(s)"=w399:dbl[], "Samples"=w397:enum16{"Single", "Multiple"})  [unwired: 1 in]
            n158 = Bundle(cluster=T20 {"Module ID"=-1, "Value(s)"=[], "Samples"=enum."Single"} ("Write AO Argument"), "Module ID"=w400, "Value(s)"=w399, "Samples"=w397) -> (w401:T20)
            n159 = call "Addressed to This Module.vi"("Module ID from Argument"=w400, "Module Admin"=w403) -> ("Addressed to this instance?"=w404:bool)  [unwired: 8 in, 1 out]
            n160 = case shown="True" w404 {
              tunnel: w405 -> [_ w409]
              tunnel: w401 -> [_ w407]
              tunnel: [_ w406] -> w398
              frame False {
              }
              frame True {
                n161 = call-poly <vilib>:"Delacor_lib_QMH_Enqueue Message (poly).vi"("Message Data"=w407, "Message"="Write AO", "Message Queue in"=w409) -> ("error out"=w406:errorcluster)  [unwired: 7 in, 1 out]
              }
            }
          }
          event User Event {
            # "Another Module called the \"Validate connection\" API Method."
            n162 = event-data() -> ("Module ID"=w413:i32, "Wait Notifier"=w411:refnum<notifier>, "wait for reply"=w410:bool)  [unwired: 1 in]
            n163 = Bundle(cluster=T21 {"Module ID"=-1, "Wait Notifier"=refnum, "wait for reply"=FALSE} ("Validate connection Argument"), "Module ID"=w413, "Wait Notifier"=w411, "wait for reply"=w410) -> (w414:T21)
            n164 = call "Addressed to This Module.vi"("Module ID from Argument"=w413, "Module Admin"=w416) -> ("Addressed to this instance?"=w417:bool)  [unwired: 8 in, 1 out]
            n165 = case shown="True" w417 {
              tunnel: w418 -> [_ w422]
              tunnel: w414 -> [_ w420]
              tunnel: [_ w419] -> w412
              frame False {
              }
              frame True {
                n166 = call-poly <vilib>:"Delacor_lib_QMH_Enqueue Message (poly).vi"("Message Data"=w420, "Message"="Validate connection", "Message Queue in"=w422) -> ("error out"=w419:errorcluster)  [unwired: 7 in, 1 out]
              }
            }
          }
          event User Event {
            # "Another Module called the \"Start continous acquisition\" API Method."
            n167 = event-data() -> ("Module ID"=w428:i32, "Task list"=w427:T4, "Timeout"=w426:i32, "Acq type"=w425:enum16{"Single", "Multiple"}, "N samples"=w424:i32)  [unwired: 1 in]
            n168 = Bundle(cluster=T22 {"Module ID"=-1, "Task list"=enum."All", "Timeout"=0, "Acq type"=enum."Single", "N samples"=0, "Data in"=variant} ("Start continous acquisition Argument"), "Module ID"=w428, "Task list"=w427, "Timeout"=w426, "Acq type"=w425, "N samples"=w424) -> (w429:T22)  [unwired: 1 in]
            n169 = call "Addressed to This Module.vi"("Module ID from Argument"=w428, "Module Admin"=w431) -> ("Addressed to this instance?"=w432:bool)  [unwired: 8 in, 1 out]
            n170 = case shown="True" w432 {
              tunnel: w433 -> [_ w437]
              tunnel: w429 -> [_ w435]
              tunnel: [_ w434] -> w423
              frame False {
              }
              frame True {
                n171 = call-poly <vilib>:"Delacor_lib_QMH_Enqueue Message (poly).vi"("Message Data"=w435, "Message"="Start continous acquisition", "Message Queue in"=w437) -> ("error out"=w434:errorcluster)  [unwired: 7 in, 1 out]
              }
            }
          }
          event User Event {
            # "Another Module called the \"Stop continuous acquisition\" API Method."
            n172 = event-data() -> ("Module ID"=w440:i32, "Boolean"=w439:bool)  [unwired: 1 in]
            n173 = Bundle(cluster=T23 {"Module ID"=-1, "Boolean"=FALSE} ("Stop continuous acquisition Argument"), "Module ID"=w440, "Boolean"=w439) -> (w441:T23)
            n174 = call "Addressed to This Module.vi"("Module ID from Argument"=w440, "Module Admin"=w443) -> ("Addressed to this instance?"=w444:bool)  [unwired: 8 in, 1 out]
            n175 = case shown="True" w444 {
              tunnel: w445 -> [_ w449]
              tunnel: w441 -> [_ w447]
              tunnel: [_ w446] -> w438
              frame False {
              }
              frame True {
                n176 = call-poly <vilib>:"Delacor_lib_QMH_Enqueue Message (poly).vi"("Message Data"=w447, "Message"="Stop continuous acquisition", "Message Queue in"=w449) -> ("error out"=w446:errorcluster)  [unwired: 7 in, 1 out]
              }
            }
          }
          event User Event {
            # "Another Module called the \"Create DO channel\" API Method."
            n177 = event-data() -> ("Module ID"=w453:i32, "lines"=w452:tag, "Channel name"=w451:string)  [unwired: 1 in]
            n178 = Bundle(cluster=T24 {"Module ID"=-1, "lines"="", "Channel name"=""} ("Create DO channel (new) Argument"), "Module ID"=w453, "lines"=w452, "Channel name"=w451) -> (w454:T24)
            n179 = call "Addressed to This Module.vi"("Module ID from Argument"=w453, "Module Admin"=w456) -> ("Addressed to this instance?"=w457:bool)  [unwired: 8 in, 1 out]
            n180 = case shown="True" w457 {
              tunnel: w458 -> [_ w462]
              tunnel: w454 -> [_ w460]
              tunnel: [_ w459] -> w450
              frame False {
              }
              frame True {
                n181 = call-poly <vilib>:"Delacor_lib_QMH_Enqueue Message (poly).vi"("Message Data"=w460, "Message"="Create DO channel", "Message Queue in"=w462) -> ("error out"=w459:errorcluster)  [unwired: 7 in, 1 out]
              }
            }
          }
          event User Event {
            # "Another Module called the \"Create CI channel\" API Method."
            n182 = event-data() -> ("Module ID"=w467:i32, "Physical channel"=w466:string, "Channel name"=w465:string, "Channel config"=w464:T36)  [unwired: 1 in]
            n183 = Bundle(cluster=T25 {"Module ID"=-1, "Physical channel"="", "Channel name"="", "Channel config"={"Initial count"=0, "Count direction"=10128, "Edge"=10280}} ("Create CI channel Argument"), "Module ID"=w467, "Physical channel"=w466, "Channel name"=w465, "Channel config"=w464) -> (w468:T25)
            n184 = call "Addressed to This Module.vi"("Module ID from Argument"=w467, "Module Admin"=w470) -> ("Addressed to this instance?"=w471:bool)  [unwired: 8 in, 1 out]
            n185 = case shown="True" w471 {
              tunnel: w472 -> [_ w476]
              tunnel: w468 -> [_ w474]
              tunnel: [_ w473] -> w463
              frame False {
              }
              frame True {
                n186 = call-poly <vilib>:"Delacor_lib_QMH_Enqueue Message (poly).vi"("Message Data"=w474, "Message"="Create CI channel", "Message Queue in"=w476) -> ("error out"=w473:errorcluster)  [unwired: 7 in, 1 out]
              }
            }
          }
          event User Event {
            # "Another Module called the \"Read CI\" API Method."
            n187 = event-data() -> ("Module ID"=w481:i32, "Samples"=w480:enum16{"Single", "Multiple"}, "Wait Notifier"=w479:refnum<notifier>, "wait for reply"=w478:bool)  [unwired: 1 in]
            n188 = Bundle(cluster=T26 {"Module ID"=-1, "Samples"=enum."Single", "Wait Notifier"=refnum, "wait for reply"=FALSE} ("Read CI Argument"), "Module ID"=w481, "Samples"=w480, "Wait Notifier"=w479, "wait for reply"=w478) -> (w482:T26)
            n189 = call "Addressed to This Module.vi"("Module ID from Argument"=w481, "Module Admin"=w484) -> ("Addressed to this instance?"=w485:bool)  [unwired: 8 in, 1 out]
            n190 = case shown="True" w485 {
              tunnel: w486 -> [_ w490]
              tunnel: w482 -> [_ w488]
              tunnel: [_ w487] -> w477
              frame False {
              }
              frame True {
                n191 = call-poly <vilib>:"Delacor_lib_QMH_Enqueue Message (poly).vi"("Message Data"=w488, "Message"="Read CI", "Message Queue in"=w490) -> ("error out"=w487:errorcluster)  [unwired: 7 in, 1 out]
              }
            }
          }
        }
        n192 = call-dynamic "Delacor_lib_QMH_Error Handler - Event Handling Loop.vi"("error in"=w169, "Message Queue in"=w163) -> ("dup error in"=w168:errorcluster)  [unwired: 8 in, 1 out]
      }
      n193 = while {
        tunnel: w37 -> [w495]
        shift-right: [w499] -> _
        shift-left: T5 {"Status"="", "DO task"="", "DI task"="", "AO task"="", "AI task"="", "Device name"="", "CI task"="", "CO task"=""} ("Data Cluster") -> [w500]
        tunnel: w41 -> [w503]
        tunnel: [w501] -> w43
        tunnel: w36 -> [w493]
        tunnel: [w492] -> w35
        tunnel: w28 -> [w491]
        stop <- w498 stop-if-true
        # "Message Handling Loop"
        n194 = call-dynamic "Delacor_lib_QMH_Dequeue Message.vi"("error in"=w503, "Message Queue in"=w495) -> ("error out"=w502:errorcluster, "Message Data"=w496:variant, "Message"=w497:string, "Message Queue out"=w494:refnum<class "Delacor_lib_QMH_Message Queue.lvclass">)  [unwired: 6 in]
        n195 = case "DQMH_MESSAGE_CASES" shown="\"Validate connection\"" w497 {
          selector: w497 -> [_ _ _ _ _ _ _ _ _ _ _ _ _ _ _ _ _ _ _ w1115 _ _ _ _]
          tunnel: w494 -> [w510 _ _ _ _ _ _ _ _ _ _ _ _ _ _ _ _ w1072 w1106 _ _ _ _ _]
          tunnel: w502 -> [w526 w547 w563 w581 w600 w778 w860 w881 w906 w931 w956 w967 w989 w1015 w1034 w1057 w1070 w1081 w1111 w1117 w1146 w1180 w1199 w1216]
          tunnel: [w511 w547 w556 w567 w588 w771 w840 w861 w886 w911 w943 w958 w980 w1006 w1028 w1048 w1070 w1077 w1109 w1118 w1137 w1171 w1193 w1207] -> w504
          tunnel: w500 -> [w508 w534 w559 w572 w595 w774 w850 w866 w884 w909 w934 w961 w978 w1004 w1027 w1046 w1069 w1076 w1096 w1116 w1136 w1167 w1198 w1202]
          tunnel: [w507 w533 w558 w572 w595 w774 w848 w864 w883 w908 w932 w961 w978 w1004 w1027 w1046 w1069 w1076 w1096 w1116 w1136 w1167 w1198 w1202] -> w499
          tunnel: [_ _ _ _ _ _ _ _ _ _ _ _ _ _ _ _ _ _ w1105 _ _ _ _ _] -> w498
          tunnel: w496 -> [_ _ w562 w579 w598 w777 w859 w880 w905 w930 w954 w965 w987 w1013 w1033 w1055 _ w1075 w1103 _ w1144 w1179 w1197 w1214]
          tunnel: w493 -> [w505 _ _ _ _ _ w844 w868 w892 w914 w937 _ _ _ _ _ _ w1074 w1099 w1113 _ w1164 _ w1205]
          tunnel: [_ _ _ _ _ _ _ _ _ _ _ _ _ _ _ _ _ _ w1101 _ _ _ _ _] -> w492
          tunnel: w491 -> [_ _ _ _ _ _ _ _ _ _ _ _ _ _ _ _ _ _ _ _ _ w1170 w1192 _]
          frame "Initialize" {
            w506 = "Initial Message" ("Initial Message")
            # "Initialize - Any operation that needs to be done before the module can receive messages. Synchronize Caller Events.vi will inform Start Module.vi that the module has launched and is ready to receive messages. Module Did Init.vi will broadcast that the module initialized."
            n196 = call "Synchronize Caller Events.vi"("error in (no error)"=w526, "Module Admin"=w505) -> ("error out"=w525:errorcluster, "Module Admin out"=w514:refnum<class "Delacor_lib_QMH_Cloneable Module Admin.lvclass">)  [unwired: 8 in]
            n197 = property class="Mod Admin"(reference=w514) -> ("Accessors:Module ID"=w516:i32, "Accessors:External Launch"=w515:bool)  [unwired: 1 in, 2 out]
            n198 = property on="Pane" class="Pane"("Origin"=T27 {"Horizontal"=0, "Vertical"=0}) -> ()  [unwired: 2 in, 2 out]
            n199 = call "Module Name--constant.vi"("Module ID"=w516) -> ("Module Name"=w522:string)  [unwired: 10 in]
            n200 = property class="VI"("Front Panel.Title"=w522) -> (reference out=w524:refnum<vi>, error out=w528:errorcluster)  [unwired: 2 in]
            n201 = Select(t=T28."Hidden" ("State"), s=w515, f=T28."Standard" ("State")) -> (s? t:f=w519:T28)
            n202 = call "Module Name--constant.vi"("Module ID"=w516) -> ("Module Name"=w517:string)  [unwired: 10 in]
            n203 = call "Module Did Init.vi"("error in (no error)"=w525, "Initialized?"=TRUE, "Origin"=w517, "Module ID"=w516) -> ("error out"=w512:errorcluster)  [unwired: 7 in]
            n204 = invoke class="VI" method="FP.Open"(reference=w524, error in=w528, "State"=w519) -> (reference out=w523:refnum<vi>, error out=w527:errorcluster)  [unwired: 2 in, 3 out]
            n205 = Bundle By Name(cluster=w508, "Status"=w506) -> (w507:T5)
            n206 = invoke class="VI" method="FP.Center"(reference=w523, error in=w527) -> ()  [unwired: 1 in, 3 out]
            n207 = call-poly <vilib>:"Delacor_lib_QMH_Enqueue Message (poly).vi"("error in"=w512, "Message"="Create tasks", "Message Queue in"=w510) -> ("error out"=w511:errorcluster)  [unwired: 7 in, 1 out]
            "Status" <- w506
          }
          frame "Create tasks" {
            n208 = call <vilib>:"Create NI GUID.vi"() -> ("NI GUID"=w546:string)
            n209 = for {
              tunnel: w546 -> [w551]
              tunnel: " %s" ("format string") -> [w550]
              tunnel: string[] ["DO task", "DI task", "AO task", "AI task", "CI task", "CO task"] ("new task name") -> [w549] mode=indexing
              tunnel: [w548] -> w539 mode=indexing
              n210 = Format Into String(format string=w550, initial string=w549, w551) -> (resulting string=w548:string)  [unwired: 1 in, 1 out]
            }
            n211 = Index Array(array=w539) -> (element #1=w535:string, element #2=w536:string, element #3=w537:string, element #4=w538:string, element #5=w532:string, element #6=w529:string)  [unwired: 6 in]
            n212 = call <vilib>:"DAQmx Create Task.vi"("new task name"=w535) -> ("task out"=w545:refnum<k21>)  [unwired: 13 in, 1 out]
            n213 = call <vilib>:"DAQmx Create Task.vi"("new task name"=w536) -> ("task out"=w544:refnum<k21>)  [unwired: 13 in, 1 out]
            n214 = call <vilib>:"DAQmx Create Task.vi"("new task name"=w537) -> ("task out"=w543:refnum<k21>)  [unwired: 13 in, 1 out]
            n215 = call <vilib>:"DAQmx Create Task.vi"("new task name"=w538) -> ("task out"=w542:refnum<k21>)  [unwired: 13 in, 1 out]
            n216 = call <vilib>:"DAQmx Create Task.vi"("new task name"=w532) -> ("task out"=w531:refnum<k21>)  [unwired: 13 in, 1 out]
            n217 = call <vilib>:"DAQmx Create Task.vi"("new task name"=w529) -> ("task out"=w530:refnum<k21>)  [unwired: 13 in, 1 out]
            n218 = Bundle By Name(cluster=w534, "DO task"=w545, "DI task"=w544, "AO task"=w543, "AI task"=w542, "CI task"=w531, "CO task"=w530) -> (w533:T5)
          }
          frame "Set device ID" {
            # "Set the device identifier to be managed internally by the module."
            n219 = Variant To Data(error in=w563, type=T8 {"Module ID"=-1, "Device ID"=""} ("Set device ID Argument"), Variant=w562) -> (data=w560:T8, error out=w557:errorcluster)
            n220 = Unbundle By Name(w560) -> ("Device ID"=w552:tag, "Module ID"=w555:i32)
            n221 = Bundle By Name(cluster=w559, "Device name"=w552) -> (w558:T5)
            n222 = Format Into String(format string="Device ID set to %s.", w552) -> (resulting string=w553:string)  [unwired: 2 in, 1 out]
            n223 = call "Status Updated.vi"("error in (no error)"=w557, "Status"=w553, "Module ID"=w555) -> ("error out"=w556:errorcluster)  [unwired: 8 in]
          }
          frame "Get channel list" {
            # "Request to read all available channels from the specified device."
            n224 = Variant To Data(error in=w581, type=T9 {"Module ID"=-1, "Wait Notifier"=refnum, "wait for reply"=FALSE} ("Get channel list Argument"), Variant=w579) -> (data=w577:T9, error out=w580:errorcluster)
            n225 = Unbundle By Name(w572) -> ("Device name"=w571:tag)
            n226 = Unbundle By Name(w577) -> ("Wait Notifier"=w576:refnum<notifier>, "wait for reply"=w575:bool, "Module ID"=w566:i32)
            n227 = call "Get Channels.vi"("ActiveDev"=w571) -> ("error out"=w570:errorcluster, "Available channels"=w564:string[][], "Available channels out"=w569:i32)  [unwired: 8 in]
            n228 = Bundle By Name(cluster=T29 {"Available channels"=0, "error"={"status"=FALSE, "code"=0, "source"=""}, "Available channels 2"=[]} ("Get channel list (Reply Payload)"), "Available channels"=w569, "Available channels 2"=w564, "error"=w570) -> (w574:T29)
            n229 = Merge Errors(w580, w570) -> (w568:errorcluster)
            n230 = case shown="True" w575 {
              tunnel: w576 -> [_ w583]
              tunnel: w574 -> [_ w582]
              frame False {
              }
              frame True {
                n231 = Send Notification(notification=w582, notifier=w583) -> ()  [unwired: 1 in, 2 out]
              }
            }
            n232 = call "Status Updated.vi"("error in (no error)"=w568, "Status"="Channel list updated.", "Module ID"=w566) -> ("error out"=w567:errorcluster)  [unwired: 8 in]
          }
          frame "Start task" {
            # "Request to start all existing channels for the local task."
            n233 = Variant To Data(error in=w600, type=T10 {"Module ID"=-1, "Task list"=enum."All"} ("Start task Argument"), Variant=w598) -> (data=w596:T10, error out=w599:errorcluster)
            n234 = Unbundle By Name(w595) -> ("DO task"=w594:refnum<k21>, "DI task"=w593:refnum<k21>, "AO task"=w592:refnum<k21>, "AI task"=w591:refnum<k21>, "CI task"=w585:refnum<k21>, "CO task"=w584:refnum<k21>)
            n235 = Unbundle By Name(w596) -> ("Task list"=w586:T4, "Module ID"=w587:i32)
            n236 = Build Array(w594, w593, w592, w591, w585, w584) -> (w589:refnum<k21>[])
            n237 = case shown="\"CI task\"" w586 {
              tunnel: [w603 w625 w648 w671 w694 w717 w740] -> w590
              tunnel: w589 -> [w602 w628 w651 w674 w697 w720 w743]
              tunnel: w587 -> [w601 w626 w649 w672 w695 w718 w741]
              frame "All", Default {
                n238 = for {
                  tunnel: [w606] -> w603
                  tunnel: w602 -> [w608] mode=indexing
                  tunnel: w601 -> [w604]
                  n239 = call <vilib>:"DAQmx Start Task.vi"("task/channels in"=w608) -> ("task out"=w605:refnum<k21>, "error out"=w607:errorcluster)  [unwired: 13 in]
                  n240 = case shown="No Error" w607 {
                    selector: w607 -> [w613 w616 w619]
                    tunnel: [w614 w617 w623] -> w606
                    tunnel: w605 -> [w611 _ _]
                    tunnel: w604 -> [w609 _ w621]
                    frame No Error {
                      n241 = Format Into String(format string="Task %s started successfuly." ("Status"), w611) -> (resulting string=w610:string)  [unwired: 2 in, 1 out]
                      n242 = call "Status Updated.vi"("error in (no error)"=w613, "Status"=w610, "Module ID"=w609) -> ("error out"=w614:errorcluster)  [unwired: 8 in]
                    }
                    frame Error {
                      # "Task has no channels"
                      n243 = call <vilib>:"Clear Errors.vi"("error in (no error)"=w616, "specific error code to clear (0: all)"=-200478) -> ("error out"=w617:errorcluster)  [unwired: 4 in, 1 out]
                    }
                    frame Default {
                      # "Unknown error"
                      n244 = call <vilib>:"Clear Errors.vi"("error in (no error)"=w619) -> ("error out"=w624:errorcluster)  [unwired: 5 in, 1 out]
                      n245 = Unbundle By Name(w619) -> ("code"=w618:i32)
                      n246 = Format Into String(format string="Unknown error while starting task. Error code: %d." ("Status"), w618) -> (resulting string=w622:string)  [unwired: 2 in, 1 out]
                      n247 = call "Status Updated.vi"("error in (no error)"=w624, "Status"=w622, "Module ID"=w621) -> ("error out"=w623:errorcluster)  [unwired: 8 in]
                    }
                  }
                }
              }
              frame "DO task" {
                n248 = Index Array(array=w628) -> (element=w627:refnum<k21>)  [unwired: 1 in]
                n249 = call <vilib>:"DAQmx Start Task.vi"("task/channels in"=w627) -> ("task out"=w630:refnum<k21>, "error out"=w629:errorcluster)  [unwired: 13 in]
                n250 = case shown="No Error" w629 {
                  selector: w629 -> [w635 w638 w641]
                  tunnel: [w636 w639 w645] -> w625
                  tunnel: w630 -> [w633 _ _]
                  tunnel: w626 -> [w631 _ w643]
                  frame No Error {
                    n251 = Format Into String(format string="Task %s started successfuly." ("Status"), w633) -> (resulting string=w632:string)  [unwired: 2 in, 1 out]
                    n252 = call "Status Updated.vi"("error in (no error)"=w635, "Status"=w632, "Module ID"=w631) -> ("error out"=w636:errorcluster)  [unwired: 8 in]
                  }
                  frame Error {
                    # "Task has no channels"
                    n253 = call <vilib>:"Clear Errors.vi"("error in (no error)"=w638, "specific error code to clear (0: all)"=-200478) -> ("error out"=w639:errorcluster)  [unwired: 4 in, 1 out]
                  }
                  frame Default {
                    # "Unknown error"
                    n254 = call <vilib>:"Clear Errors.vi"("error in (no error)"=w641) -> ("error out"=w646:errorcluster)  [unwired: 5 in, 1 out]
                    n255 = Unbundle By Name(w641) -> ("code"=w640:i32)
                    n256 = Format Into String(format string="Unknown error while starting task. Error code: %d." ("Status"), w640) -> (resulting string=w644:string)  [unwired: 2 in, 1 out]
                    n257 = call "Status Updated.vi"("error in (no error)"=w646, "Status"=w644, "Module ID"=w643) -> ("error out"=w645:errorcluster)  [unwired: 8 in]
                  }
                }
              }
              frame "DI task" {
                n258 = Index Array(array=w651, index=1) -> (element=w650:refnum<k21>)
                n259 = call <vilib>:"DAQmx Start Task.vi"("task/channels in"=w650) -> ("task out"=w653:refnum<k21>, "error out"=w652:errorcluster)  [unwired: 13 in]
                n260 = case shown="No Error" w652 {
                  selector: w652 -> [w658 w661 w664]
                  tunnel: [w659 w662 w668] -> w648
                  tunnel: w653 -> [w656 _ _]
                  tunnel: w649 -> [w654 _ w666]
                  frame No Error {
                    n261 = Format Into String(format string="Task %s started successfuly." ("Status"), w656) -> (resulting string=w655:string)  [unwired: 2 in, 1 out]
                    n262 = call "Status Updated.vi"("error in (no error)"=w658, "Status"=w655, "Module ID"=w654) -> ("error out"=w659:errorcluster)  [unwired: 8 in]
                  }
                  frame Error {
                    # "Task has no channels"
                    n263 = call <vilib>:"Clear Errors.vi"("error in (no error)"=w661, "specific error code to clear (0: all)"=-200478) -> ("error out"=w662:errorcluster)  [unwired: 4 in, 1 out]
                  }
                  frame Default {
                    # "Unknown error"
                    n264 = call <vilib>:"Clear Errors.vi"("error in (no error)"=w664) -> ("error out"=w669:errorcluster)  [unwired: 5 in, 1 out]
                    n265 = Unbundle By Name(w664) -> ("code"=w663:i32)
                    n266 = Format Into String(format string="Unknown error while starting task. Error code: %d." ("Status"), w663) -> (resulting string=w667:string)  [unwired: 2 in, 1 out]
                    n267 = call "Status Updated.vi"("error in (no error)"=w669, "Status"=w667, "Module ID"=w666) -> ("error out"=w668:errorcluster)  [unwired: 8 in]
                  }
                }
              }
              frame "AO task" {
                n268 = Index Array(array=w674, index=2) -> (element=w673:refnum<k21>)
                n269 = call <vilib>:"DAQmx Start Task.vi"("task/channels in"=w673) -> ("task out"=w676:refnum<k21>, "error out"=w675:errorcluster)  [unwired: 13 in]
                n270 = case shown="No Error" w675 {
                  selector: w675 -> [w681 w684 w687]
                  tunnel: [w682 w685 w691] -> w671
                  tunnel: w676 -> [w679 _ _]
                  tunnel: w672 -> [w677 _ w689]
                  frame No Error {
                    n271 = Format Into String(format string="Task %s started successfuly." ("Status"), w679) -> (resulting string=w678:string)  [unwired: 2 in, 1 out]
                    n272 = call "Status Updated.vi"("error in (no error)"=w681, "Status"=w678, "Module ID"=w677) -> ("error out"=w682:errorcluster)  [unwired: 8 in]
                  }
                  frame Error {
                    # "Task has no channels"
                    n273 = call <vilib>:"Clear Errors.vi"("error in (no error)"=w684, "specific error code to clear (0: all)"=-200478) -> ("error out"=w685:errorcluster)  [unwired: 4 in, 1 out]
                  }
                  frame Default {
                    # "Unknown error"
                    n274 = call <vilib>:"Clear Errors.vi"("error in (no error)"=w687) -> ("error out"=w692:errorcluster)  [unwired: 5 in, 1 out]
                    n275 = Unbundle By Name(w687) -> ("code"=w686:i32)
                    n276 = Format Into String(format string="Unknown error while starting task. Error code: %d." ("Status"), w686) -> (resulting string=w690:string)  [unwired: 2 in, 1 out]
                    n277 = call "Status Updated.vi"("error in (no error)"=w692, "Status"=w690, "Module ID"=w689) -> ("error out"=w691:errorcluster)  [unwired: 8 in]
                  }
                }
              }
              frame "AI task" {
                n278 = Index Array(array=w697, index=3) -> (element=w696:refnum<k21>)
                n279 = call <vilib>:"DAQmx Start Task.vi"("task/channels in"=w696) -> ("task out"=w699:refnum<k21>, "error out"=w698:errorcluster)  [unwired: 13 in]
                n280 = case shown="No Error" w698 {
                  selector: w698 -> [w704 w707 w710]
                  tunnel: [w705 w708 w714] -> w694
                  tunnel: w699 -> [w702 _ _]
                  tunnel: w695 -> [w700 _ w712]
                  frame No Error {
                    n281 = Format Into String(format string="Task %s started successfuly." ("Status"), w702) -> (resulting string=w701:string)  [unwired: 2 in, 1 out]
                    n282 = call "Status Updated.vi"("error in (no error)"=w704, "Status"=w701, "Module ID"=w700) -> ("error out"=w705:errorcluster)  [unwired: 8 in]
                  }
                  frame Error {
                    # "Task has no channels"
                    n283 = call <vilib>:"Clear Errors.vi"("error in (no error)"=w707, "specific error code to clear (0: all)"=-200478) -> ("error out"=w708:errorcluster)  [unwired: 4 in, 1 out]
                  }
                  frame Default {
                    # "Unknown error"
                    n284 = call <vilib>:"Clear Errors.vi"("error in (no error)"=w710) -> ("error out"=w715:errorcluster)  [unwired: 5 in, 1 out]
                    n285 = Unbundle By Name(w710) -> ("code"=w709:i32)
                    n286 = Format Into String(format string="Unknown error while starting task. Error code: %d." ("Status"), w709) -> (resulting string=w713:string)  [unwired: 2 in, 1 out]
                    n287 = call "Status Updated.vi"("error in (no error)"=w715, "Status"=w713, "Module ID"=w712) -> ("error out"=w714:errorcluster)  [unwired: 8 in]
                  }
                }
              }
              frame "CI task" {
                n288 = Index Array(array=w720, index=4) -> (element=w719:refnum<k21>)
                n289 = call <vilib>:"DAQmx Start Task.vi"("task/channels in"=w719) -> ("task out"=w722:refnum<k21>, "error out"=w721:errorcluster)  [unwired: 13 in]
                n290 = case shown="Default" w721 {
                  selector: w721 -> [w727 w730 w733]
                  tunnel: [w728 w731 w737] -> w717
                  tunnel: w722 -> [w725 _ _]
                  tunnel: w718 -> [w723 _ w735]
                  frame No Error {
                    n291 = Format Into String(format string="Task %s started successfuly." ("Status"), w725) -> (resulting string=w724:string)  [unwired: 2 in, 1 out]
                    n292 = call "Status Updated.vi"("error in (no error)"=w727, "Status"=w724, "Module ID"=w723) -> ("error out"=w728:errorcluster)  [unwired: 8 in]
                  }
                  frame Error {
                    # "Task has no channels"
                    n293 = call <vilib>:"Clear Errors.vi"("error in (no error)"=w730, "specific error code to clear (0: all)"=-200478) -> ("error out"=w731:errorcluster)  [unwired: 4 in, 1 out]
                  }
                  frame Default {
                    # "Unknown error"
                    n294 = call <vilib>:"Clear Errors.vi"("error in (no error)"=w733) -> ("error out"=w738:errorcluster)  [unwired: 5 in, 1 out]
                    n295 = Unbundle By Name(w733) -> ("code"=w732:i32)
                    n296 = Format Into String(format string="Unknown error while starting task. Error code: %d." ("Status"), w732) -> (resulting string=w736:string)  [unwired: 2 in, 1 out]
                    n297 = call "Status Updated.vi"("error in (no error)"=w738, "Status"=w736, "Module ID"=w735) -> ("error out"=w737:errorcluster)  [unwired: 8 in]
                  }
                }
              }
              frame "CO task" {
                n298 = Index Array(array=w743, index=5) -> (element=w742:refnum<k21>)
                n299 = call <vilib>:"DAQmx Start Task.vi"("task/channels in"=w742) -> ("task out"=w745:refnum<k21>, "error out"=w744:errorcluster)  [unwired: 13 in]
                n300 = case shown="No Error" w744 {
                  selector: w744 -> [w750 w753 w756]
                  tunnel: [w751 w754 w760] -> w740
                  tunnel: w745 -> [w748 _ _]
                  tunnel: w741 -> [w746 _ w758]
                  frame No Error {
                    n301 = Format Into String(format string="Task %s started successfuly." ("Status"), w748) -> (resulting string=w747:string)  [unwired: 2 in, 1 out]
                    n302 = call "Status Updated.vi"("error in (no error)"=w750, "Status"=w747, "Module ID"=w746) -> ("error out"=w751:errorcluster)  [unwired: 8 in]
                  }
                  frame Error {
                    # "Task has no channels"
                    n303 = call <vilib>:"Clear Errors.vi"("error in (no error)"=w753, "specific error code to clear (0: all)"=-200478) -> ("error out"=w754:errorcluster)  [unwired: 4 in, 1 out]
                  }
                  frame Default {
                    # "Unknown error"
                    n304 = call <vilib>:"Clear Errors.vi"("error in (no error)"=w756) -> ("error out"=w761:errorcluster)  [unwired: 5 in, 1 out]
                    n305 = Unbundle By Name(w756) -> ("code"=w755:i32)
                    n306 = Format Into String(format string="Unknown error while starting task. Error code: %d." ("Status"), w755) -> (resulting string=w759:string)  [unwired: 2 in, 1 out]
                    n307 = call "Status Updated.vi"("error in (no error)"=w761, "Status"=w759, "Module ID"=w758) -> ("error out"=w760:errorcluster)  [unwired: 8 in]
                  }
                }
              }
            }
            n308 = Merge Errors(w599, w590) -> (w588:errorcluster)
          }
          frame "Stop task" {
            # "Request to stop all channels within the local task."
            n309 = Variant To Data(error in=w778, type=T11 {"Module ID"=-1, "Task list"=enum."All"} ("Stop task Argument"), Variant=w777) -> (data=w775:T11, error out=w773:errorcluster)
            n310 = Unbundle By Name(w774) -> ("DO task"=w770:refnum<k21>, "DI task"=w769:refnum<k21>, "AO task"=w768:refnum<k21>, "AI task"=w767:refnum<k21>, "CI task"=w763:refnum<k21>, "CO task"=w762:refnum<k21>)
            n311 = Unbundle By Name(w775) -> ("Task list"=w766:T4, "Module ID"=w764:i32)
            n312 = Build Array(w770, w769, w768, w767, w763, w762) -> (w765:refnum<k21>[])
            n313 = case shown="\"CO task\"" w766 {
              tunnel: [w780 w793 w799 w806 w816 w825 w834] -> w772
              tunnel: w765 -> [w783 w794 w796 w805 w814 w823 w832]
              tunnel: w764 -> [w781 w791 w798 w807 w815 w824 w833]
              frame "All", Default {
                n314 = for {
                  tunnel: w783 -> [w786] mode=indexing
                  shift-right: [w785] -> w779
                  shift-left: _ -> [w784]
                  n315 = call <vilib>:"DAQmx Stop Task.vi"("task/channels in"=w786, "error in"=w784) -> ("error out"=w785:errorcluster)  [unwired: 12 in, 1 out]
                }
                n316 = call "Status Updated.vi"("error in (no error)"=w779, "Status"="All tasks stopped. Standing by.", "Module ID"=w781) -> ("error out"=w780:errorcluster)  [unwired: 8 in]
              }
              frame "DO task" {
                n317 = Index Array(array=w794) -> (element=w790:refnum<k21>)  [unwired: 1 in]
                n318 = call <vilib>:"DAQmx Stop Task.vi"("task/channels in"=w790) -> ("task out"=w787:refnum<k21>, "error out"=w792:errorcluster)  [unwired: 13 in]
                n319 = Format Into String(format string="Task %s stopped. Standing by." ("Status"), w787) -> (resulting string=w788:string)  [unwired: 2 in, 1 out]
                n320 = call "Status Updated.vi"("error in (no error)"=w792, "Status"=w788, "Module ID"=w791) -> ("error out"=w793:errorcluster)  [unwired: 8 in]
              }
              frame "DI task" {
                n321 = Index Array(array=w796, index=1) -> (element=w797:refnum<k21>)
                n322 = call <vilib>:"DAQmx Stop Task.vi"("task/channels in"=w797) -> ("task out"=w800:refnum<k21>, "error out"=w803:errorcluster)  [unwired: 13 in]
                n323 = Format Into String(format string="Task %s stopped. Standing by." ("Status"), w800) -> (resulting string=w801:string)  [unwired: 2 in, 1 out]
                n324 = call "Status Updated.vi"("error in (no error)"=w803, "Status"=w801, "Module ID"=w798) -> ("error out"=w799:errorcluster)  [unwired: 8 in]
              }
              frame "AO task" {
                n325 = Index Array(array=w805, index=2) -> (element=w811:refnum<k21>)
                n326 = call <vilib>:"DAQmx Stop Task.vi"("task/channels in"=w811) -> ("task out"=w808:refnum<k21>, "error out"=w812:errorcluster)  [unwired: 13 in]
                n327 = Format Into String(format string="Task %s stopped. Standing by." ("Status"), w808) -> (resulting string=w809:string)  [unwired: 2 in, 1 out]
                n328 = call "Status Updated.vi"("error in (no error)"=w812, "Status"=w809, "Module ID"=w807) -> ("error out"=w806:errorcluster)  [unwired: 8 in]
              }
              frame "AI task" {
                n329 = Index Array(array=w814, index=3) -> (element=w819:refnum<k21>)
                n330 = call <vilib>:"DAQmx Stop Task.vi"("task/channels in"=w819) -> ("task out"=w821:refnum<k21>, "error out"=w818:errorcluster)  [unwired: 13 in]
                n331 = Format Into String(format string="Task %s stopped. Standing by." ("Status"), w821) -> (resulting string=w820:string)  [unwired: 2 in, 1 out]
                n332 = call "Status Updated.vi"("error in (no error)"=w818, "Status"=w820, "Module ID"=w815) -> ("error out"=w816:errorcluster)  [unwired: 8 in]
              }
              frame "CI task" {
                n333 = Index Array(array=w823, index=4) -> (element=w828:refnum<k21>)
                n334 = call <vilib>:"DAQmx Stop Task.vi"("task/channels in"=w828) -> ("task out"=w830:refnum<k21>, "error out"=w827:errorcluster)  [unwired: 13 in]
                n335 = Format Into String(format string="Task %s stopped. Standing by." ("Status"), w830) -> (resulting string=w829:string)  [unwired: 2 in, 1 out]
                n336 = call "Status Updated.vi"("error in (no error)"=w827, "Status"=w829, "Module ID"=w824) -> ("error out"=w825:errorcluster)  [unwired: 8 in]
              }
              frame "CO task" {
                n337 = Index Array(array=w832, index=5) -> (element=w837:refnum<k21>)
                n338 = call <vilib>:"DAQmx Stop Task.vi"("task/channels in"=w837) -> ("task out"=w839:refnum<k21>, "error out"=w836:errorcluster)  [unwired: 13 in]
                n339 = Format Into String(format string="Task %s stopped. Standing by." ("Status"), w839) -> (resulting string=w838:string)  [unwired: 2 in, 1 out]
                n340 = call "Status Updated.vi"("error in (no error)"=w836, "Status"=w838, "Module ID"=w833) -> ("error out"=w834:errorcluster)  [unwired: 8 in]
              }
            }
            n341 = Merge Errors(w773, w772) -> (w771:errorcluster)
          }
          frame "Create DO channel" {
            # "Creates a new digital output with a single or multiple channels."
            n342 = Variant To Data(error in=w860, type=T24 {"Module ID"=-1, "lines"="", "Channel name"=""} ("Create DO channel (new) Argument"), Variant=w859) -> (data=w857:T24, error out=w842:errorcluster)
            n343 = Unbundle By Name(w850) -> ("DO task"=w853:refnum<k21>, "Device name"=w854:tag)
            n344 = property class="Mod Admin"(reference=w844) -> ("Accessors:Module ID"=w843:i32)  [unwired: 1 in, 2 out]
            n345 = Unbundle By Name(w857) -> ("lines"=w855:tag, "Channel name"=w846:string)
            n346 = Format Into String(format string="%s/%s", w854, w855) -> (resulting string=w847:string)  [unwired: 2 in, 1 out]
            n347 = call-poly <vilib>:"DAQmx Create Virtual Channel.vi"("task in"=w853, "lines"=w847, "name to assign"=w846) -> ("task out"=w849:refnum<k21>, "error out"=w845:errorcluster)  [unwired: 11 in]
            n348 = Format Into String(format string="Channel %s created. Standing by.", w846) -> (resulting string=w851:string)  [unwired: 2 in, 1 out]
            n349 = Bundle By Name(cluster=w850, "DO task"=w849) -> (w848:T5)
            n350 = call "Status Updated.vi"("error in (no error)"=w845, "Status"=w851, "Module ID"=w843) -> ("error out"=w841:errorcluster)  [unwired: 8 in]
            n351 = Merge Errors(w842, w841) -> (w840:errorcluster)
          }
          frame "Create DI channel" {
            # "Request to create a digital input channel(s)."
            n352 = Variant To Data(error in=w881, type=T13 {"Module ID"=-1, "Physical channel"="", "Channel name"=""} ("Create DI channel Argument"), Variant=w880) -> (data=w878:T13, error out=w871:errorcluster)
            n353 = property class="Mod Admin"(reference=w868) -> ("Accessors:Module ID"=w867:i32)  [unwired: 1 in, 2 out]
            n354 = Unbundle By Name(w866) -> ("DI task"=w875:refnum<k21>, "Device name"=w876:tag)
            n355 = Unbundle By Name(w878) -> ("Physical channel"=w874:string, "Channel name"=w873:string)
            n356 = Format Into String(format string="%s/%s", w876, w874) -> (resulting string=w870:string)  [unwired: 2 in, 1 out]
            n357 = call-poly <vilib>:"DAQmx Create Virtual Channel.vi"("task in"=w875, "lines"=w870, "name to assign"=w873) -> ("task out"=w865:refnum<k21>, "error out"=w863:errorcluster)  [unwired: 11 in]
            n358 = Format Into String(format string="Channel %s created. Standing by.", w870) -> (resulting string=w869:string)  [unwired: 2 in, 1 out]
            n359 = Bundle By Name(cluster=w866, "DI task"=w865) -> (w864:T5)
            n360 = call "Status Updated.vi"("error in (no error)"=w863, "Status"=w869, "Module ID"=w867) -> ("error out"=w862:errorcluster)  [unwired: 8 in]
            n361 = Merge Errors(w871, w862) -> (w861:errorcluster)
          }
          frame "Create AI channel" {
            # "Request to create an analog input channel in the selected channel."
            n362 = Variant To Data(error in=w906, type=T16 {"Module ID"=-1, "Physical channel"="", "Channel name"="", "Config params"={"input terminal configuration"=-1, "minimum value"=-5.0, "maximum value"=5.0}} ("Create AI channel Argument"), Variant=w905) -> (data=w903:T16, error out=w887:errorcluster)
            n363 = Unbundle By Name(w903) -> ("Config params"=w901:T35, "Physical channel"=w896:string, "Channel name"=w897:string)
            n364 = property class="Mod Admin"(reference=w892) -> ("Accessors:Module ID"=w891:i32)  [unwired: 1 in, 2 out]
            n365 = Unbundle By Name(w884) -> ("AI task"=w895:refnum<k21>, "Device name"=w894:tag)
            n366 = Unbundle By Name(w901) -> ("input terminal configuration"=w900:i32, "minimum value"=w899:dbl, "maximum value"=w898:dbl)
            n367 = Format Into String(format string="%s/%s", w894, w896) -> (resulting string=w889:string)  [unwired: 2 in, 1 out]
            n368 = call-poly <vilib>:"DAQmx Create Virtual Channel.vi"("task in"=w895, "maximum value"=w898, "minimum value"=w899, "input terminal configuration"=w900, "physical channels"=w889, "name to assign"=w897) -> ("task out"=w882:refnum<k21>, "error out"=w893:errorcluster)  [unwired: 8 in]
            n369 = Format Into String(format string="Channel %s created. Standing by.", w889) -> (resulting string=w888:string)  [unwired: 2 in, 1 out]
            n370 = Bundle By Name(cluster=w884, "AI task"=w882) -> (w883:T5)
            n371 = call "Status Updated.vi"("error in (no error)"=w893, "Status"=w888, "Module ID"=w891) -> ("error out"=w885:errorcluster)  [unwired: 8 in]
            n372 = Merge Errors(w887, w885) -> (w886:errorcluster)
          }
          frame "Create AO channel" {
            # "Request to create single or multiple analog output channel (s)."
            n373 = Variant To Data(error in=w931, type=T18 {"Module ID"=-1, "Physical channel"="", "Channel name"="", "Config params"={"Terminal configuration"=-1, "min value"=-5.0, "max value"=5.0}} ("Create AO channel Argument"), Variant=w930) -> (data=w928:T18, error out=w912:errorcluster)
            n374 = property class="Mod Admin"(reference=w914) -> ("Accessors:Module ID"=w913:i32)  [unwired: 1 in, 2 out]
            n375 = Unbundle By Name(w928) -> ("Config params"=w922:T19, "Physical channel"=w925:string, "Channel name"=w923:string)
            n376 = Unbundle By Name(w909) -> ("AO task"=w924:refnum<k21>, "Device name"=w926:tag)
            n377 = Unbundle By Name(w922) -> ("Terminal configuration"=w921:i32, "min value"=w920:dbl, "max value"=w919:dbl)
            n378 = Format Into String(format string="%s/%s", w926, w925) -> (resulting string=w917:string)  [unwired: 2 in, 1 out]
            n379 = call-poly <vilib>:"DAQmx Create Virtual Channel.vi"("task in"=w924, "maximum value"=w919, "minimum value"=w920, "output terminal configuration"=w921, "physical channels"=w917, "name to assign"=w923) -> ("task out"=w907:refnum<k21>, "error out"=w916:errorcluster)  [unwired: 8 in]
            n380 = Format Into String(format string="Channel %s created. Standing by.", w917) -> (resulting string=w915:string)  [unwired: 2 in, 1 out]
            n381 = Bundle By Name(cluster=w909, "AO task"=w907) -> (w908:T5)
            n382 = call "Status Updated.vi"("error in (no error)"=w916, "Status"=w915, "Module ID"=w913) -> ("error out"=w910:errorcluster)  [unwired: 8 in]
            n383 = Merge Errors(w912, w910) -> (w911:errorcluster)
          }
          frame "Create CI channel" {
            # "Request to create a counter input channel."
            n384 = Variant To Data(error in=w956, type=T25 {"Module ID"=-1, "Physical channel"="", "Channel name"="", "Channel config"={"Initial count"=0, "Count direction"=10128, "Edge"=10280}} ("Create CI channel Argument"), Variant=w954) -> (data=w952:T25, error out=w955:errorcluster)
            n385 = property class="Mod Admin"(reference=w937) -> ("Accessors:Module ID"=w936:i32)  [unwired: 1 in, 2 out]
            n386 = Unbundle By Name(w952) -> ("Channel config"=w947:T36, "Physical channel"=w949:string, "Channel name"=w948:string)
            n387 = Unbundle By Name(w934) -> ("CI task"=w942:refnum<k21>, "Device name"=w950:tag)
            n388 = Unbundle By Name(w947) -> ("Edge"=w946:i32, "Count direction"=w945:i32, "Initial count"=w944:u32)
            n389 = Format Into String(format string="%s/%s", w950, w949) -> (resulting string=w940:string)  [unwired: 2 in, 1 out]
            n390 = call-poly <vilib>:"DAQmx Create Virtual Channel.vi"("task in"=w942, "initial count"=w944, "count direction"=w945, "edge"=w946, "counter"=w940, "name to assign"=w948) -> ("task out"=w933:refnum<k21>, "error out"=w939:errorcluster)  [unwired: 8 in]
            n391 = Format Into String(format string="Channel %s created. Standing by.", w940) -> (resulting string=w938:string)  [unwired: 2 in, 1 out]
            n392 = Bundle By Name(cluster=w934, "CI task"=w933) -> (w932:T5)
            n393 = call "Status Updated.vi"("error in (no error)"=w939, "Status"=w938, "Module ID"=w936) -> ("error out"=w935:errorcluster)  [unwired: 8 in]
            n394 = Merge Errors(w935, w955) -> (w943:errorcluster)
          }
          frame "Write DO" {
            # "Request to write to a single or multiple digital output channels."
            n395 = Variant To Data(error in=w967, type=T12 {"Module ID"=-1, "Samples"=enum."Single", "Data"=[]} ("Write DO Argument"), Variant=w965) -> (data=w963:T12, error out=w966:errorcluster)
            n396 = Unbundle By Name(w961) -> ("DO task"=w960:refnum<k21>)
            n397 = Unbundle By Name(w963) -> ("Data"=w959:bool[], "Samples"=w962:enum16{"Single", "Multiple"})
            n398 = case shown="\"Single\", Default" w962 {
              tunnel: w960 -> [w970 w974]
              tunnel: w959 -> [w969 w972]
              tunnel: [w971 w973] -> w957
              frame "Single", Default {
                n399 = Index Array(array=w969) -> (element=w968:bool)  [unwired: 1 in]
                n400 = call-poly <vilib>:"DAQmx Write.vi"("task/channels in"=w970, "data"=w968) -> ("error out"=w971:errorcluster)  [unwired: 11 in, 2 out]
              }
              frame "Multiple" {
                n401 = call-poly <vilib>:"DAQmx Write.vi"("task/channels in"=w974, "data"=w972) -> ("error out"=w973:errorcluster)  [unwired: 11 in, 2 out]
              }
            }
            n402 = Merge Errors(w966, w957) -> (w958:errorcluster)
          }
          frame "Read DI" {
            # "Request to read one or multiple digital inputs."
            n403 = Variant To Data(error in=w989, type=T14 {"Module ID"=-1, "Samples"=enum."Single", "Wait Notifier"=refnum, "wait for reply"=FALSE} ("Read DI Argument"), Variant=w987) -> (data=w985:T14, error out=w988:errorcluster)
            n404 = Unbundle By Name(w985) -> ("Wait Notifier"=w984:refnum<notifier>, "wait for reply"=w983:bool, "Samples"=w979:enum16{"Single", "Multiple"})
            n405 = Unbundle By Name(w978) -> ("DI task"=w977:refnum<k21>)
            n406 = case shown="\"Multiple\"" w979 {
              tunnel: w977 -> [w993 w998]
              tunnel: [w991 w996] -> w976
              tunnel: [w990 w997] -> w975
              frame "Single", Default {
                n407 = call-poly <vilib>:"DAQmx Read.vi"("task/channels in"=w993) -> ("data"=w992:bool, "error out"=w990:errorcluster)  [unwired: 12 in, 1 out]
                n408 = Build Array(w992) -> (w991:bool[])
              }
              frame "Multiple" {
                n409 = call-poly <vilib>:"DAQmx Read.vi"("task/channels in"=w998) -> ("data"=w995:u8[], "error out"=w997:errorcluster)  [unwired: 12 in, 1 out]
                n410 = Index Array(array=w995) -> (element=w994:u8)  [unwired: 1 in]
                n411 = Number To Boolean Array(number=w994) -> (Boolean array=w996:bool[])
              }
            }
            n412 = Merge Errors(w988, w975) -> (w980:errorcluster)
            n413 = Bundle By Name(cluster=T30 {"Data"=[], "error"={"status"=FALSE, "code"=0, "source"=""}} ("Read DI (Reply Payload)"), "Data"=w976, "error"=w975) -> (w982:T30)
            n414 = case shown="True" w983 {
              tunnel: w984 -> [_ w1000]
              tunnel: w982 -> [_ w999]
              frame False {
              }
              frame True {
                n415 = Send Notification(notification=w999, notifier=w1000) -> ()  [unwired: 1 in, 2 out]
              }
            }
          }
          frame "Read AI" {
            # "Request to read single or multiple analog inputs."
            n416 = Variant To Data(error in=w1015, type=T17 {"Module ID"=-1, "Samples"=enum."Single", "Wait Notifier"=refnum, "wait for reply"=FALSE} ("Read AI Argument"), Variant=w1013) -> (data=w1011:T17, error out=w1014:errorcluster)
            n417 = Unbundle By Name(w1011) -> ("Wait Notifier"=w1010:refnum<notifier>, "wait for reply"=w1009:bool, "Samples"=w1005:enum16{"Single", "Multiple"})
            n418 = Unbundle By Name(w1004) -> ("AI task"=w1003:refnum<k21>)
            n419 = case shown="\"Single\"" w1005 {
              tunnel: w1003 -> [w1018 w1022]
              tunnel: [w1017 w1019] -> w1002
              tunnel: [w1016 w1021] -> w1001
              frame "Multiple", Default {
                n420 = call-poly <vilib>:"DAQmx Read.vi"("task/channels in"=w1018) -> ("data"=w1017:dbl[], "error out"=w1016:errorcluster)  [unwired: 12 in, 1 out]
              }
              frame "Single" {
                n421 = call-poly <vilib>:"DAQmx Read.vi"("task/channels in"=w1022) -> ("data"=w1020:dbl, "error out"=w1021:errorcluster)  [unwired: 12 in, 1 out]
                n422 = Build Array(w1020) -> (w1019:dbl[])
              }
            }
            n423 = Bundle By Name(cluster=T31 {"Data"=[], "error"={"status"=FALSE, "code"=0, "source"=""}} ("Read AI (Reply Payload)"), "Data"=w1002, "error"=w1001) -> (w1008:T31)
            n424 = Merge Errors(w1014, w1001) -> (w1006:errorcluster)
            n425 = case shown="True" w1009 {
              tunnel: w1010 -> [_ w1024]
              tunnel: w1008 -> [_ w1023]
              frame False {
              }
              frame True {
                n426 = Send Notification(notification=w1023, notifier=w1024) -> ()  [unwired: 1 in, 2 out]
              }
            }
          }
          frame "Write AO" {
            # "Request to write a value to a single or multiple channel (s)"
            n427 = Variant To Data(error in=w1034, type=T20 {"Module ID"=-1, "Value(s)"=[], "Samples"=enum."Single"} ("Write AO Argument"), Variant=w1033) -> (data=w1031:T20, error out=w1029:errorcluster)
            n428 = Unbundle By Name(w1027) -> ("AO task"=w1026:refnum<k21>)
            n429 = Unbundle By Name(w1031) -> ("Samples"=w1030:enum16{"Single", "Multiple"}, "Value(s)"=w1025:dbl[])
            n430 = case shown="\"Multiple\", Default" w1030 {
              tunnel: w1029 -> [w1039 w1043]
              tunnel: [w1038 w1042] -> w1028
              tunnel: w1026 -> [w1037 w1041]
              tunnel: w1025 -> [w1036 w1040]
              frame "Multiple", Default {
                n431 = Index Array(array=w1036) -> (element=w1035:dbl)  [unwired: 1 in]
                n432 = call-poly <vilib>:"DAQmx Write.vi"("task/channels in"=w1037, "data"=w1035, "error in"=w1039) -> ("error out"=w1038:errorcluster)  [unwired: 10 in, 2 out]
              }
              frame "Single" {
                n433 = call-poly <vilib>:"DAQmx Write.vi"("task/channels in"=w1041, "data"=w1040, "error in"=w1043) -> ("error out"=w1042:errorcluster)  [unwired: 10 in, 2 out]
              }
            }
          }
          frame "Get task ref" {
            # "Request to get a reference to a given task."
            n434 = Variant To Data(error in=w1057, type=T15 {"Module ID"=-1, "Task list"=enum."All", "Wait Notifier"=refnum, "wait for reply"=FALSE} ("Get task ref Argument"), Variant=w1055) -> (data=w1053:T15, error out=w1056:errorcluster)
            n435 = Unbundle By Name(w1053) -> ("Task list"=w1047:T4, "Wait Notifier"=w1052:refnum<notifier>, "wait for reply"=w1051:bool)
            n436 = case shown="\"DO task\"" w1047 {
              tunnel: w1046 -> [_ w1060 w1062 w1064 w1066]
              tunnel: [_ w1059 w1061 w1063 w1065] -> w1045
              tunnel: [errorcluster {"status"=FALSE, "code"=0, "source"=""} ("error in (no error)") _ _ _ _] -> w1044
              frame "All", Default {
              }
              frame "DO task" {
                n437 = Unbundle By Name(w1060) -> ("DO task"=w1059:refnum<k21>)
              }
              frame "DI task" {
                n438 = Unbundle By Name(w1062) -> ("DI task"=w1061:refnum<k21>)
              }
              frame "AO task" {
                n439 = Unbundle By Name(w1064) -> ("AO task"=w1063:refnum<k21>)
              }
              frame "AI task" {
                n440 = Unbundle By Name(w1066) -> ("AI task"=w1065:refnum<k21>)
              }
            }
            n441 = Bundle By Name(cluster=T32 {"DAQmx Task"="", "error"={"status"=FALSE, "code"=0, "source"=""}} ("Get task ref (Reply Payload)"), "DAQmx Task"=w1045, "error"=w1044) -> (w1050:T32)
            n442 = Merge Errors(w1056, w1044) -> (w1048:errorcluster)
            n443 = case shown="True" w1051 {
              tunnel: w1052 -> [_ w1068]
              tunnel: w1050 -> [_ w1067]
              frame False {
              }
              frame True {
                n444 = Send Notification(notification=w1067, notifier=w1068) -> ()  [unwired: 1 in, 2 out]
              }
            }
          }
          frame "---Exit and Error Handling---" {
            # "Separator - the following cases handle errors and exit messages."
          }
          frame "Error" {
            # "#CodeRecommended - If you ever change the name of this \"Error\" message, you'll need to update the name in the Check Loop Error.vi as well."
            # "#CodeRecommended - If the module is running in standalone mode (External Launch = FALSE), this code will pop up an error dialog and call the 'Exit' message if an error occurs. Add more fine-grained error handling here."
            # "Error - Check the error message data and respond accordingly. This message is sent by the \"Error Handler\" VIs at the end of each loop in this application."
            n445 = property class="Mod Admin"(reference=w1074) -> ("Accessors:External Launch"=w1073:bool, "Accessors:Module ID"=w1071:i32)  [unwired: 1 in, 2 out]
            n446 = Variant To Data(error in=w1081, type=errorcluster {"status"=FALSE, "code"=0, "source"=""} ("error constant"), Variant=w1075) -> (data=w1082:errorcluster, error out=w1079:errorcluster)
            n447 = call "Error Reported.vi"("Error"=w1082, "Module ID"=w1071) -> ()  [unwired: 9 in, 1 out]
            n448 = case shown="False" w1073 {
              tunnel: [w1087 _] -> w1078
              tunnel: w1072 -> [w1085 _]
              tunnel: w1082 -> [w1086 _]
              frame False {
                # "If the module is running standalone, then pop up an error dialog and call the \"Exit\" message."
                n449 = call <vilib>:"Simple Error Handler.vi"("error in (no error)"=w1086) -> ()  [unwired: 4 in, 5 out]
                n450 = call-poly <vilib>:"Delacor_lib_QMH_Enqueue Message (poly).vi"("Priority Message? (F)"=TRUE, "Message"="Exit", "Message Queue in"=w1085) -> ("error out"=w1087:errorcluster)  [unwired: 7 in, 1 out]
              }
              frame True {
                # "If the module was launched externally, calling the Error Reported broadcast VI is the only action performed by the \"Error\" message. The module's caller can then process the error appropriately."
              }
            }
            n451 = Merge Errors(w1079, w1078) -> (w1077:errorcluster)
            n452 = local write "error out"(w1077) -> ()
          }
          frame "Exit" {
            w1104 = 91  # 91: not all Exit messages will have an argument
            w1105 = TRUE  # Stop the VI
            # "Release the message queue reference"
            # "Exit - Exit the application."
            n453 = Variant To Data(error in=w1111, type=T7 {"Module ID"=-1, "Origin"="", "Exit via Stop Module Req?"=FALSE, "Wait for Module to stop?"=FALSE} ("Stop Argument"), Variant=w1103) -> (data=w1100:T7, error out=w1107:errorcluster)
            n454 = call <vilib>:"Clear Errors.vi"("error in (no error)"=w1107, "specific error code to clear (0: all)"=w1104) -> ("error out"=w1110:errorcluster)  [unwired: 4 in, 1 out]
            n455 = Unbundle By Name(w1096) -> ("DO task"=w1088:refnum<k21>, "DI task"=w1089:refnum<k21>, "AO task"=w1090:refnum<k21>, "AI task"=w1095:refnum<k21>)
            n456 = call-dynamic "Delacor_lib_QMH_Release Message Queue.vi"("error in"=w1110, "Message Queue"=w1106) -> ("error out"=w1097:errorcluster)  [unwired: 9 in]
            n457 = control-ref of="This VI"() -> (w1098:refnum<vi>)
            n458 = call <vilib>:"DAQmx Clear Task.vi"("task in"=w1095, "error in"=w1097) -> ("error out"=w1094:errorcluster)  [unwired: 13 in]
            n459 = call "Handle Exit.vi"("Stop Argument"=w1100, "Module Admin in"=w1099, "VI reference"=w1098) -> ("error out"=w1108:errorcluster, "Wait for Stop?"=w1101:bool)  [unwired: 7 in]
            n460 = call <vilib>:"DAQmx Clear Task.vi"("task in"=w1090, "error in"=w1094) -> ("error out"=w1093:errorcluster)  [unwired: 13 in]
            n461 = call <vilib>:"DAQmx Clear Task.vi"("task in"=w1089, "error in"=w1093) -> ("error out"=w1092:errorcluster)  [unwired: 13 in]
            n462 = call <vilib>:"DAQmx Clear Task.vi"("task in"=w1088, "error in"=w1092) -> ("error out"=w1091:errorcluster)  [unwired: 13 in]
            n463 = Merge Errors(w1091, w1108) -> (w1109:errorcluster)
          }
          frame Default {
            # "'Default' case only runs if there is a message that isn't defined in any of the other cases.  Output a programming error."
            n464 = property class="Mod Admin"(reference=w1113) -> ("Accessors:Module ID"=w1112:i32)  [unwired: 1 in, 2 out]
            n465 = call "Module Name--constant.vi"("Module ID"=w1112) -> ("Module Name"=w1114:string)  [unwired: 10 in]
            n466 = xnode "Error Ring"("parameter 0"=w1115, "parameter 1"=w1114) -> ("error out"=w1119:errorcluster)
            n467 = Merge Errors(w1117, w1119) -> (w1118:errorcluster)
          }
          frame "Validate connection" {
            # "Request to validate correct connection to device. Call after the Set device ID event."
            n468 = property class="DAQmx System"() -> (error out=w1135:errorcluster, "DevNames"=w1132:tag[])  [unwired: 2 in, 1 out]
            n469 = Variant To Data(error in=w1146, type=T21 {"Module ID"=-1, "Wait Notifier"=refnum, "wait for reply"=FALSE} ("Validate connection Argument"), Variant=w1144) -> (data=w1142:T21, error out=w1145:errorcluster)
            n470 = Unbundle By Name(w1136) -> ("Device name"=w1131:tag)
            n471 = Unbundle By Name(w1142) -> ("Module ID"=w1133:i32, "Wait Notifier"=w1141:refnum<notifier>, "wait for reply"=w1140:bool)
            n472 = for {
              tunnel: w1132 -> [w1160] mode=indexing
              tunnel: w1131 -> [w1158]
              tunnel: [w1159] -> w1130
              tunnel: [w1158] -> w1129
              stop <- w1159 stop-if-true
              n473 = Equal?(x=w1158, y=w1160) -> (x = y?=w1159:bool)
            }
            n474 = case shown="False" w1130 {
              tunnel: w1135 -> [w1151 w1157]
              tunnel: [w1150 w1156] -> w1134
              tunnel: w1133 -> [w1149 w1154]
              tunnel: w1129 -> [_ w1153]
              tunnel: [u32 0 ("DevSerialNum") w1152] -> w1128
              frame False {
                n475 = call "Connection failed.vi"("error in"=w1151, "Connected?"=FALSE, "Module ID"=w1149) -> ("error out"=w1150:errorcluster)  [unwired: 8 in]
              }
              frame True {
                n476 = property class="DAQmx Device"("Active Device"=w1153) -> ("DevSerialNum"=w1152:u32)  [unwired: 2 in, 2 out]
                n477 = call "Device connected.vi"("error in"=w1157, "Connected?"=TRUE, "Module ID"=w1154) -> ("error out"=w1156:errorcluster)  [unwired: 8 in]
              }
            }
            n478 = Bundle By Name(cluster=T33 {"DevSerialNum"=0, "error"={"status"=FALSE, "code"=0, "source"=""}} ("Validate connection (Reply Payload)"), "DevSerialNum"=w1128, "error"=w1134) -> (w1139:T33)
            n479 = Merge Errors(w1145, w1134) -> (w1137:errorcluster)
            n480 = case shown="True" w1140 {
              tunnel: w1141 -> [_ w1162]
              tunnel: w1139 -> [_ w1161]
              frame False {
              }
              frame True {
                n481 = Send Notification(notification=w1161, notifier=w1162) -> ()  [unwired: 1 in, 2 out]
              }
            }
          }
          frame "Start continous acquisition" {
            # "Request to acquire continuously from DAQ device with a predefined Timeout period."
            n482 = Variant To Data(error in=w1180, type=T22 {"Module ID"=-1, "Task list"=enum."All", "Timeout"=0, "Acq type"=enum."Single", "N samples"=0, "Data in"=variant} ("Start continous acquisition Argument"), Variant=w1179) -> (data=w1177:T22, error out=w1172:errorcluster)
            n483 = property class="Mod Admin"(reference=w1164) -> ("Accessors:Module ID"=w1163:i32)  [unwired: 1 in, 2 out]
            n484 = Unbundle By Name(w1177) -> ("Task list"=w1168:T4, "Timeout"=w1175:i32, "Acq type"=w1174:enum16{"Single", "Multiple"}, "N samples"=w1173:i32, "Data in"=w1165:variant)
            n485 = case shown="\"DI task\"" w1168 {
              tunnel: w1167 -> [w1182 w1184 w1186 w1188 w1190]
              tunnel: [w1181 w1183 w1185 w1187 w1189] -> w1166
              frame Default {
                n486 = Unbundle By Name(w1182) -> ("DO task"=w1181:refnum<k21>)
              }
              frame "DO task" {
                n487 = Unbundle By Name(w1184) -> ("DO task"=w1183:refnum<k21>)
              }
              frame "DI task" {
                n488 = Unbundle By Name(w1186) -> ("DI task"=w1185:refnum<k21>)
              }
              frame "AO task" {
                n489 = Unbundle By Name(w1188) -> ("AO task"=w1187:refnum<k21>)
              }
              frame "AI task" {
                n490 = Unbundle By Name(w1190) -> ("AI task"=w1189:refnum<k21>)
              }
            }
            n491 = Bundle By Name(cluster=T3 {"Module ID"=0, "Task list"=enum."All", "Timeout"=0, "Acq type"=enum."Single", "Data in"=variant, "DAQmx Task"="", "N samples"=0} ("event data"), "DAQmx Task"=w1166, "Module ID"=w1163, "Task list"=w1168, "Timeout"=w1175, "Acq type"=w1174, "N samples"=w1173, "Data in"=w1165) -> (w1169:T3)
            n492 = call "Wake HL.vi"("error in (no error)"=w1172, "event data"=w1169, "User events"=w1170) -> ("error out"=w1171:errorcluster)  [unwired: 8 in]
          }
          frame "Stop continuous acquisition" {
            # "Request to stop continous acquisition made by the HL."
            n493 = Variant To Data(error in=w1199, type=T23 {"Module ID"=-1, "Boolean"=FALSE} ("Stop continuous acquisition Argument"), Variant=w1197) -> (data=w1195:T23, error out=w1194:errorcluster)
            n494 = Unbundle By Name(w1195) -> ("Boolean"=w1191:bool)  [unwired: 1 out]
            n495 = call "Sleep HL -- subVI.vi"("error in (no error)"=w1194, "User events"=w1192, "event data"=w1191) -> ("error out"=w1193:errorcluster)  [unwired: 8 in]
          }
          frame "Read CI" {
            # "Request to read the number of pulses of CI channels."
            n496 = Variant To Data(error in=w1216, type=T26 {"Module ID"=-1, "Samples"=enum."Single", "Wait Notifier"=refnum, "wait for reply"=FALSE} ("Read CI Argument"), Variant=w1214) -> (data=w1212:T26, error out=w1215:errorcluster)
            n497 = property class="Mod Admin"(reference=w1205) -> ("Accessors:Module ID"=w1206:i32)  [unwired: 1 in, 2 out]
            n498 = Unbundle By Name(w1212) -> ("Samples"=w1204:enum16{"Single", "Multiple"}, "Wait Notifier"=w1211:refnum<notifier>, "wait for reply"=w1210:bool)
            n499 = Unbundle By Name(w1202) -> ("CI task"=w1201:refnum<k21>)
            n500 = case shown="\"Multiple\"" w1204 {
              tunnel: [w1219 w1221] -> w1203
              tunnel: [w1218 w1222] -> w1200
              tunnel: w1201 -> [w1217 w1223]
              frame "Single", Default {
                n501 = call-poly <vilib>:"DAQmx Read.vi"("task/channels in"=w1217) -> ("data"=w1220:dbl, "error out"=w1218:errorcluster)  [unwired: 12 in, 1 out]
                n502 = Build Array(w1220) -> (w1219:dbl[])
              }
              frame "Multiple" {
                n503 = call-poly <vilib>:"DAQmx Read.vi"("task/channels in"=w1223) -> ("data"=w1221:dbl[], "error out"=w1222:errorcluster)  [unwired: 12 in, 1 out]
              }
            }
            n504 = Bundle By Name(cluster=T34 {"Module ID"=-1, "data"=[], "error"={"status"=FALSE, "code"=0, "source"=""}} ("Read CI (Reply Payload)"), "Module ID"=w1206, "data"=w1203, "error"=w1200) -> (w1209:T34)
            n505 = Merge Errors(w1215, w1200) -> (w1207:errorcluster)
            n506 = case "DQMH_FIRE_NOTIFIER" shown="True" w1210 {
              tunnel: w1211 -> [_ w1225]
              tunnel: w1209 -> [_ w1224]
              frame False {
              }
              frame True {
                n507 = Send Notification(notification=w1224, notifier=w1225) -> ()  [unwired: 1 in, 2 out]
              }
            }
          }
        }
        n508 = call-dynamic "Delacor_lib_QMH_Error Handler - Message Handling Loop.vi"("error in"=w504, "Message Queue in"=w494) -> ("dup error in"=w501:errorcluster)  [unwired: 8 in, 1 out]
      }
    }
    frame Error {
      n509 = call "Synchronize Caller Events.vi"("Module Admin"=w1233) -> ("Module Admin out"=w1232:refnum<class "Delacor_lib_QMH_Cloneable Module Admin.lvclass">)  [unwired: 9 in, 1 out]
      n510 = property class="Mod Admin"(reference=w1232) -> ("Accessors:Module ID"=w1231:i32)  [unwired: 1 in, 2 out]
      n511 = call-dynamic "Delacor_lib_QMH_Release Message Queue.vi"("error in"=w1230, "Message Queue"=w1228) -> ("error out"=w1229:errorcluster)  [unwired: 9 in]
      n512 = call "Module Name--constant.vi"("Module ID"=w1231) -> ("Module Name"=w1236:string)  [unwired: 10 in]
      n513 = Format Into String(format string="An error occurred during initialization. %s is no longer running.", w1236) -> (resulting string=w1234:string)  [unwired: 2 in, 1 out]
      n514 = call "Error Reported.vi"("Additional Information"=w1234, "Error"=w1229, "Module ID"=w1231) -> ()  [unwired: 8 in, 1 out]
    }
  }
  n515 = Unregister For Events(event registration refnum=w4, error in=w1) -> (error out=w3:errorcluster)
  n516 = Merge Errors(w26, w25, w3) -> (w6:errorcluster)
  n517 = call "Destroy user events.vi"("error in (no error)"=w6, "User events"=w7) -> ("error out"=w5:errorcluster)  [unwired: 9 in]
  n518 = call "Close Module.vi"("error in"=w5, "Wait for stop?"=w13, "Module Admin in"=w10) -> ("error out"=w23:errorcluster, "External Launch"=w12:bool, "Module Admin out"=w14:refnum<class "Delacor_lib_QMH_Cloneable Module Admin.lvclass">)  [unwired: 6 in]
  n519 = Unregister For Events(event registration refnum=w18, error in=w23) -> (error out=w22:errorcluster)
  "error out" <- w22
  n520 = case "External Launch?" shown="True" w12 {
    tunnel: w22 -> [_ w1238]
    frame False {
    }
    frame True {
      n521 = case shown="No Error" w1238 {
        frame No Error {
          n522 = invoke class="VI" method="FP.Close"() -> ()  [unwired: 3 in, 3 out]
        }
        frame Error {
          n523 = invoke class="VI" method="FP.Open"("Activate"=TRUE ("Activate?")) -> ()  [unwired: 4 in, 5 out]
        }
      }
    }
  }
  n524 = local write "Module Admin"(w14) -> ()
